vi "r3_stave HDI measure shih v1.vi"() -> ()   [LabVIEW 2016]
uses:
  <vilib>/Utility/file.llb/Read Delimited Spreadsheet (DBL).vi
  <vilib>/Utility/file.llb/Write Delimited Spreadsheet (DBL).vi
  Classes/Controllers/Motion/Copy of Motion Folder/Motion.lvclass
  Classes/Controllers/Camera/Copy of Controller Folder/Controller.lvclass
panel:
  in  "south - bottom right":bool
  in  "south - bottom left":bool
  in  "south - upper left":bool
  in  "north - bottom right":bool
  in  "north - bottom left":bool
  in  "north - upper left":bool
  out "txt check":dbl[][](array[numeric])
  in  "north first switch":bool
  out "position from OGP all":dbl[][][](array[numeric]) format="%#_8g"
  out "HDI-stave deviation all":dbl[][][](array[numeric]) format="%#_8g"
  out "HDI - stave deviation on time":dbl[][](array[numeric]) format="%#_8g"
  out "position from OGP on time":dbl[][](array[numeric]) format="%#_8g"
  in  "default south HDI upper left":dbl[](array[numeric])=[589.61399, 909.79853, 66.641535, 0.0001909297]
  in  "test":bool
  in  "how much HDI":i32=2
  out "bottom right":dbl[][](array[numeric]) format="%#_8g"
  out "bottom left":dbl[][](array[numeric]) format="%#_8g"
  out "top left":dbl[][](array[numeric]) format="%#_8g"
  out "HDI center position":dbl[][](array[numeric]) format="%#_8g"
  in  "default north HDI upper left":dbl[](array[numeric])=[589.67627, 676.52803, 66.636955, 0.0001904]
  in  "Default HDI size":dbl[](array[numeric])=[24.2437, 231.446, -0.099339, 0.000191129]
  out "measure times":dbl
  in  "Parking position":dbl[](array[numeric])=[625.0, 625.0, 0.0, 0.01]
  in  "measure HDI position":bool
  in  "calculate":bool
  in  "go to park":bool
  in  "stop":bool
  # "Please click the \"make north first\" before calculate\nIf there is new txt from \"Bless from OGP\", please click \"make north first\", then click the \"calculate\""
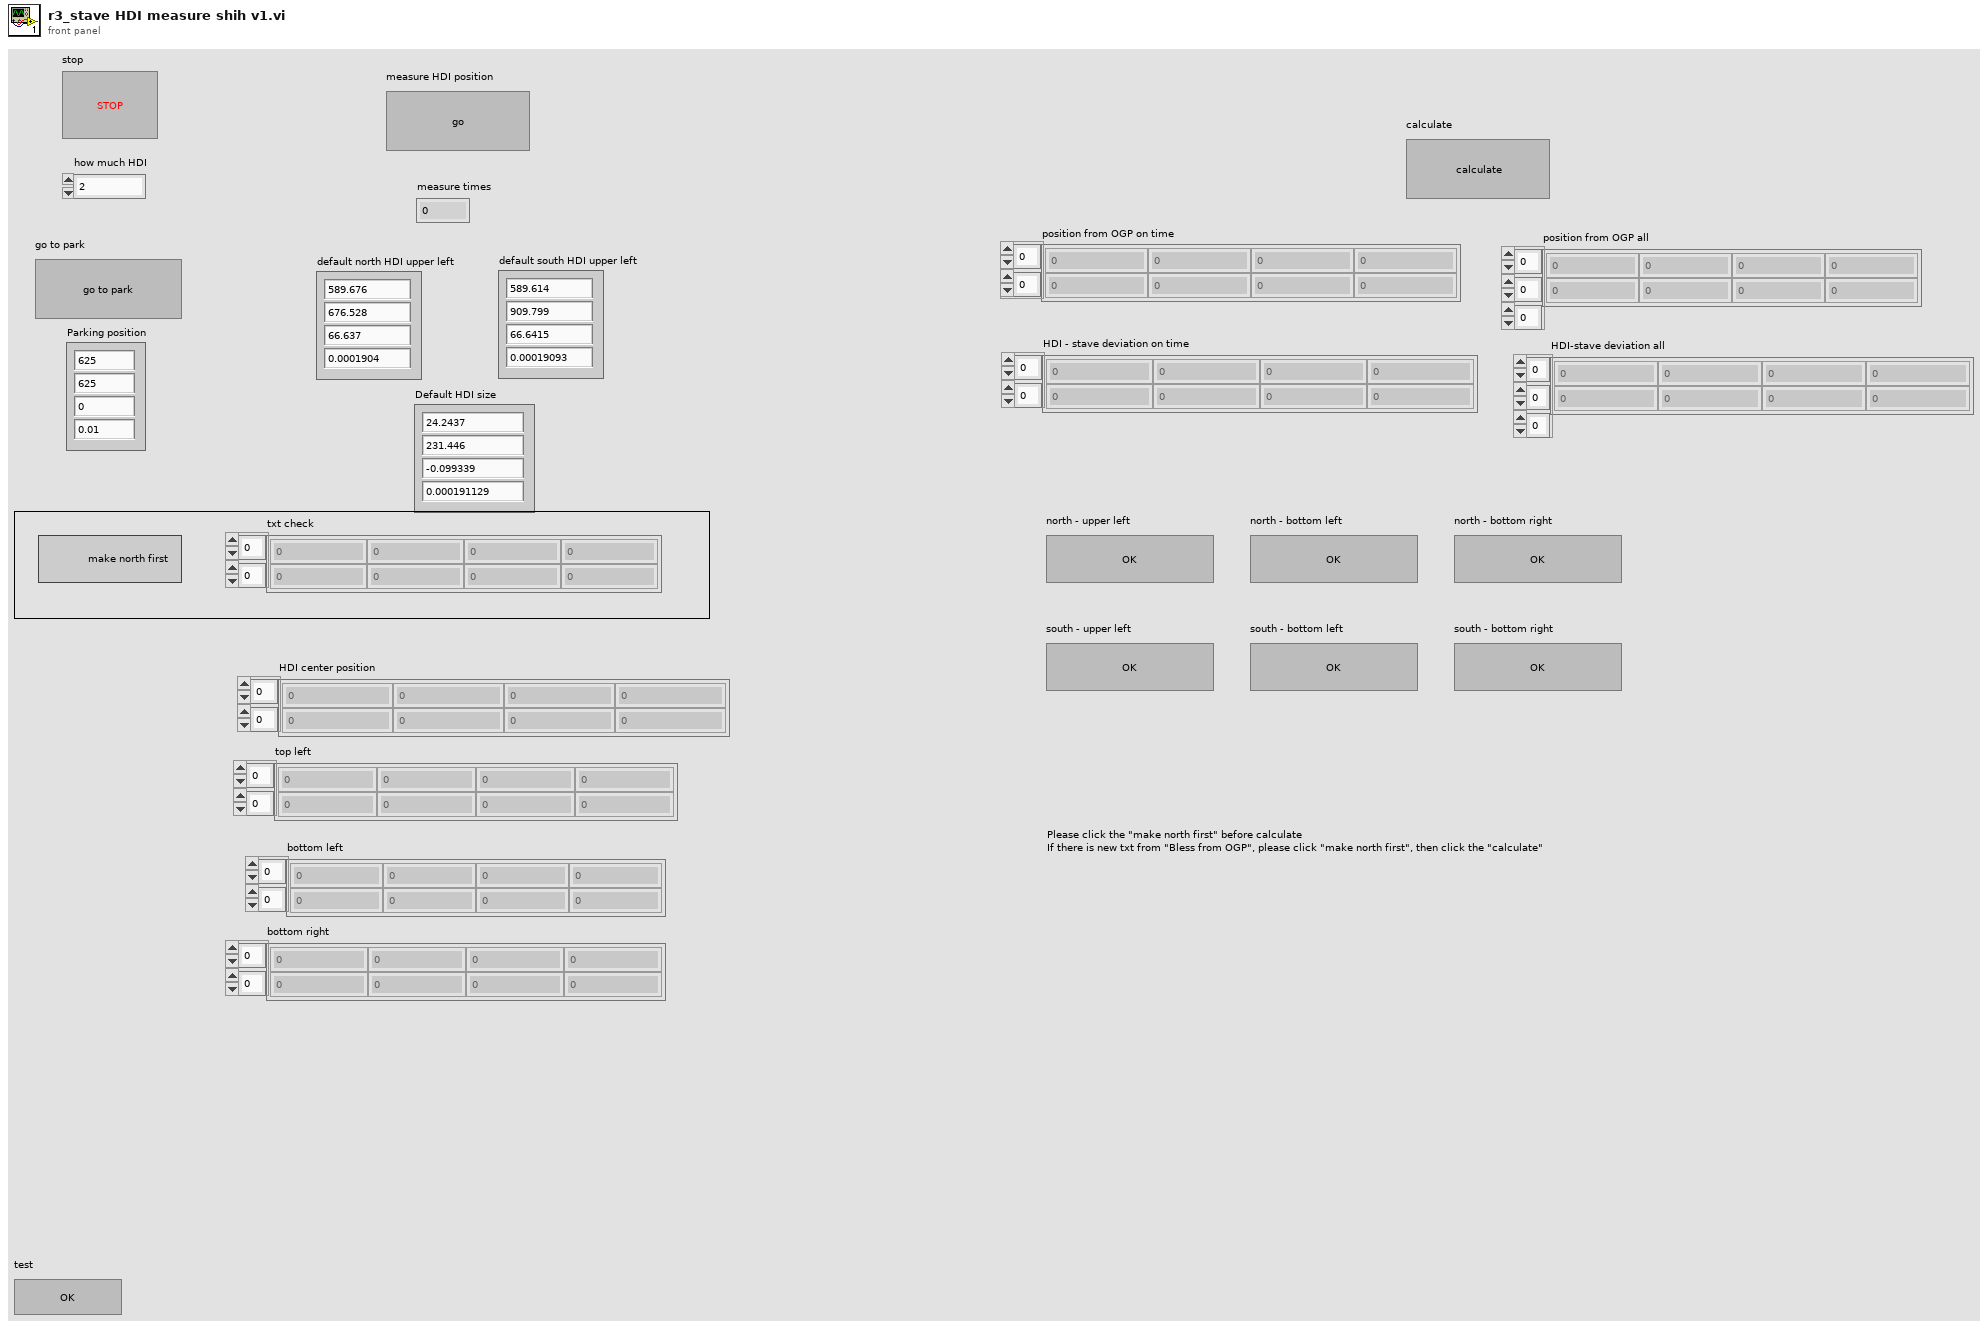
[diagram p1: front panel]
types:
  T1 = typedef "Controller.lvclass/Controllers.ctl" = cluster{"Copy of Motion.lvclass":refnum<class "Motion.lvclass">, "Copy of I-O.lvclass":refnum<class "I-O.lvclass">, "Copy of Dispenser.lvclass":refnum<class "Dispenser.lvclass">}
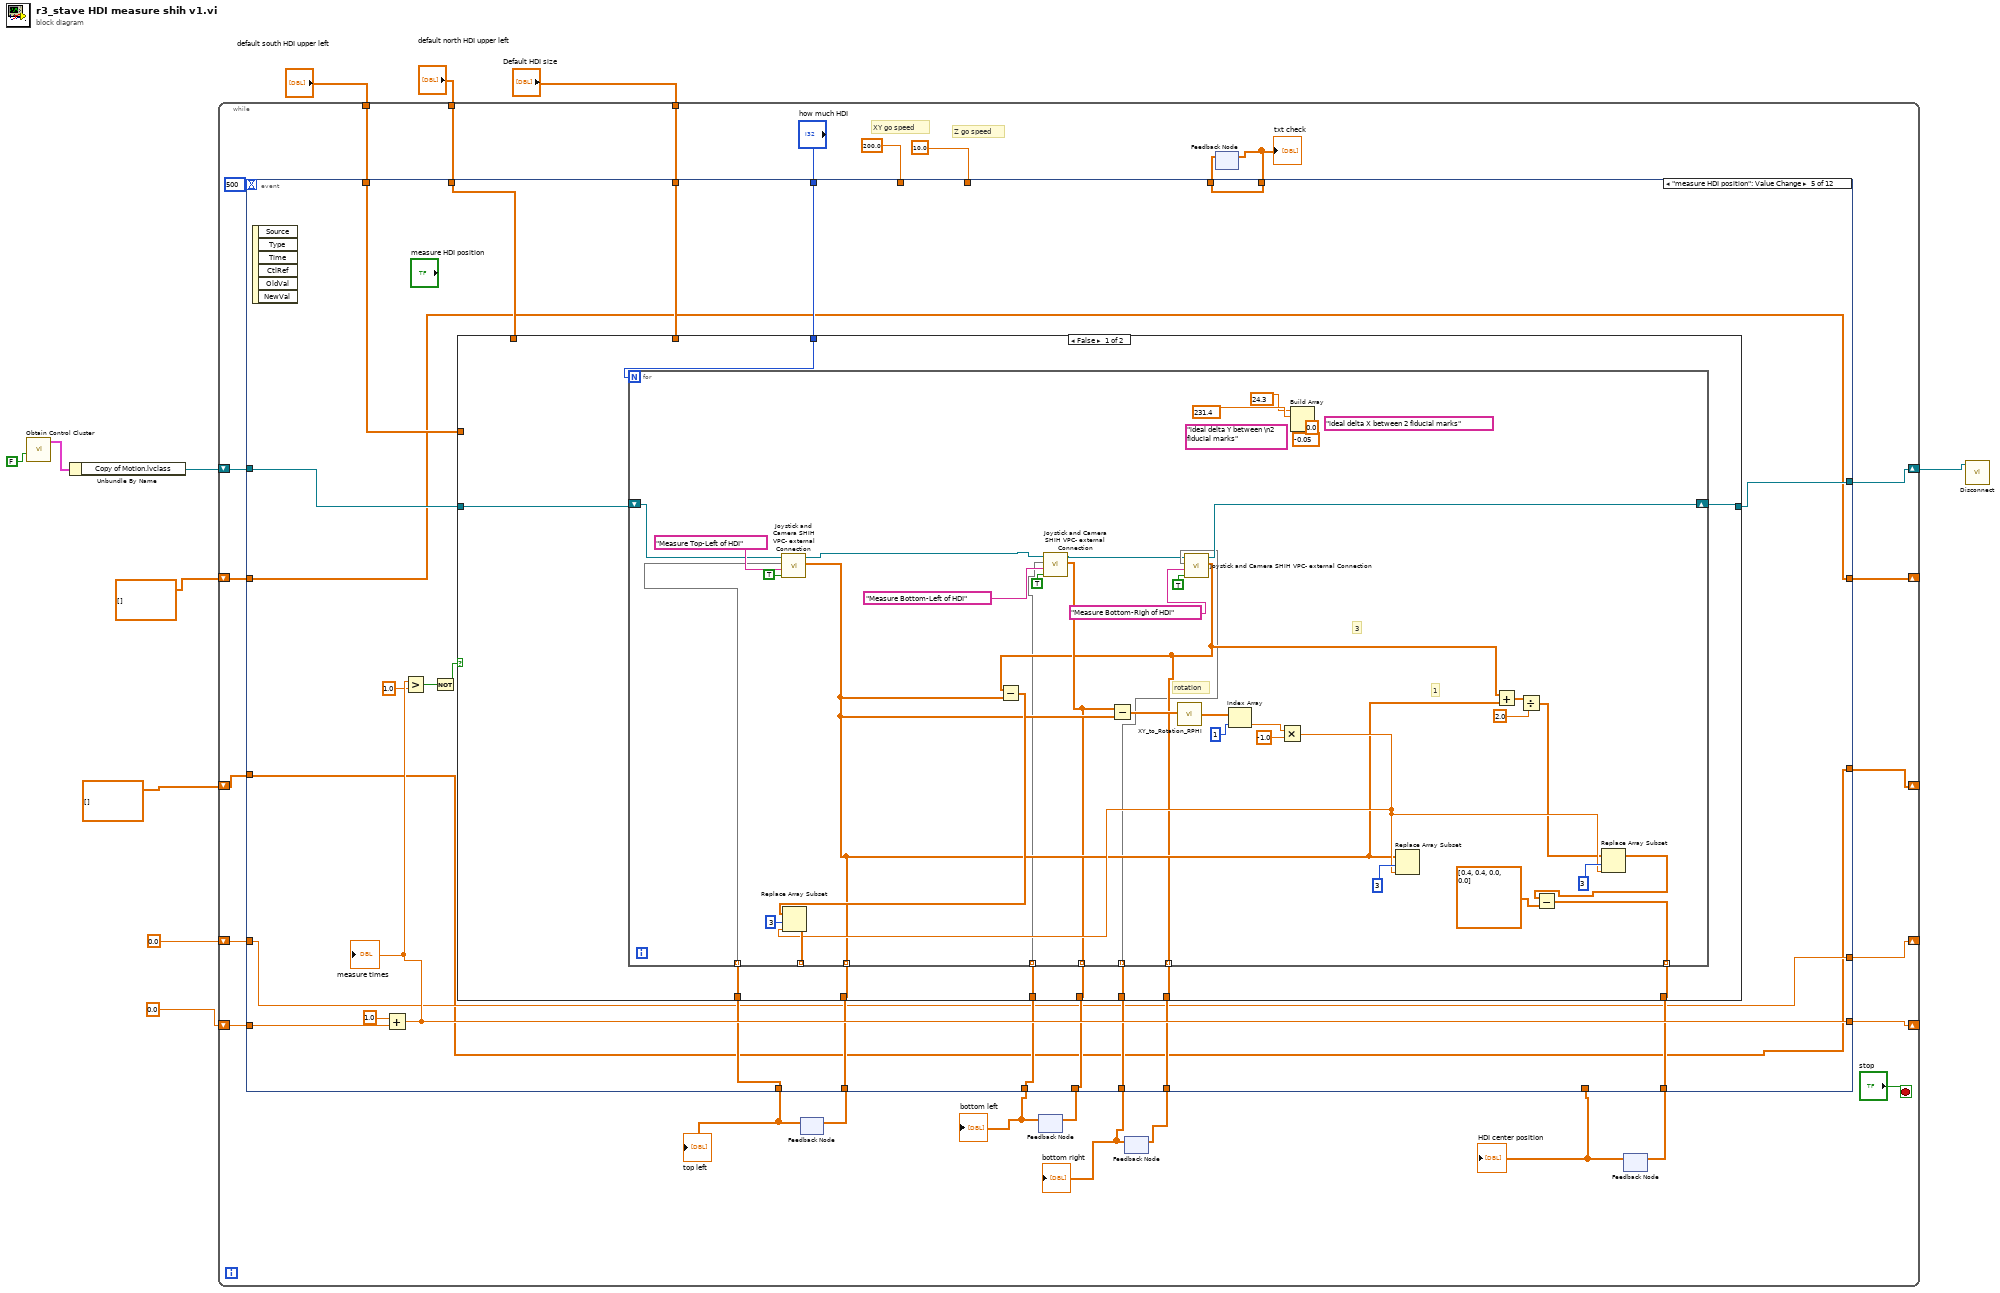
[diagram p0: block diagram]
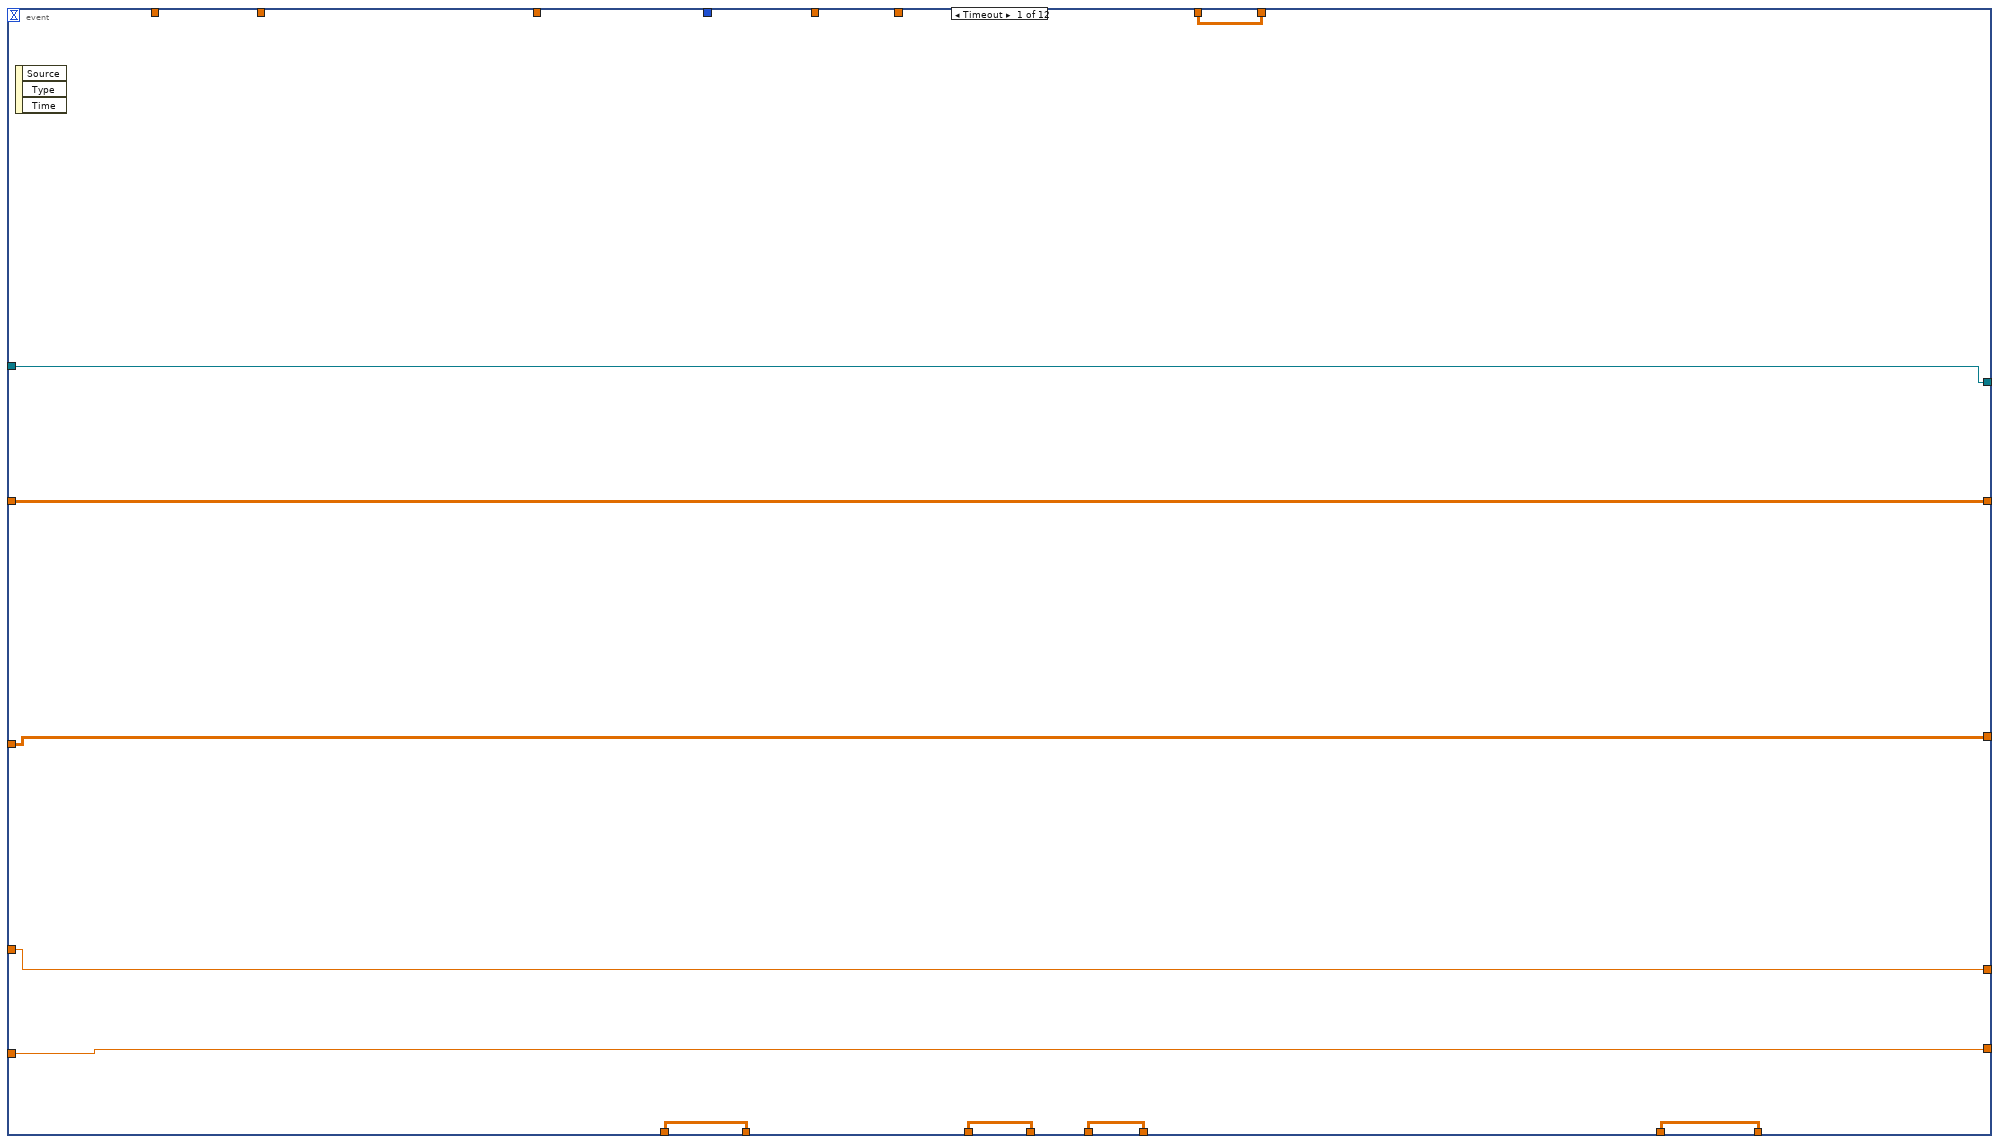
[diagram p2: hidden frame]
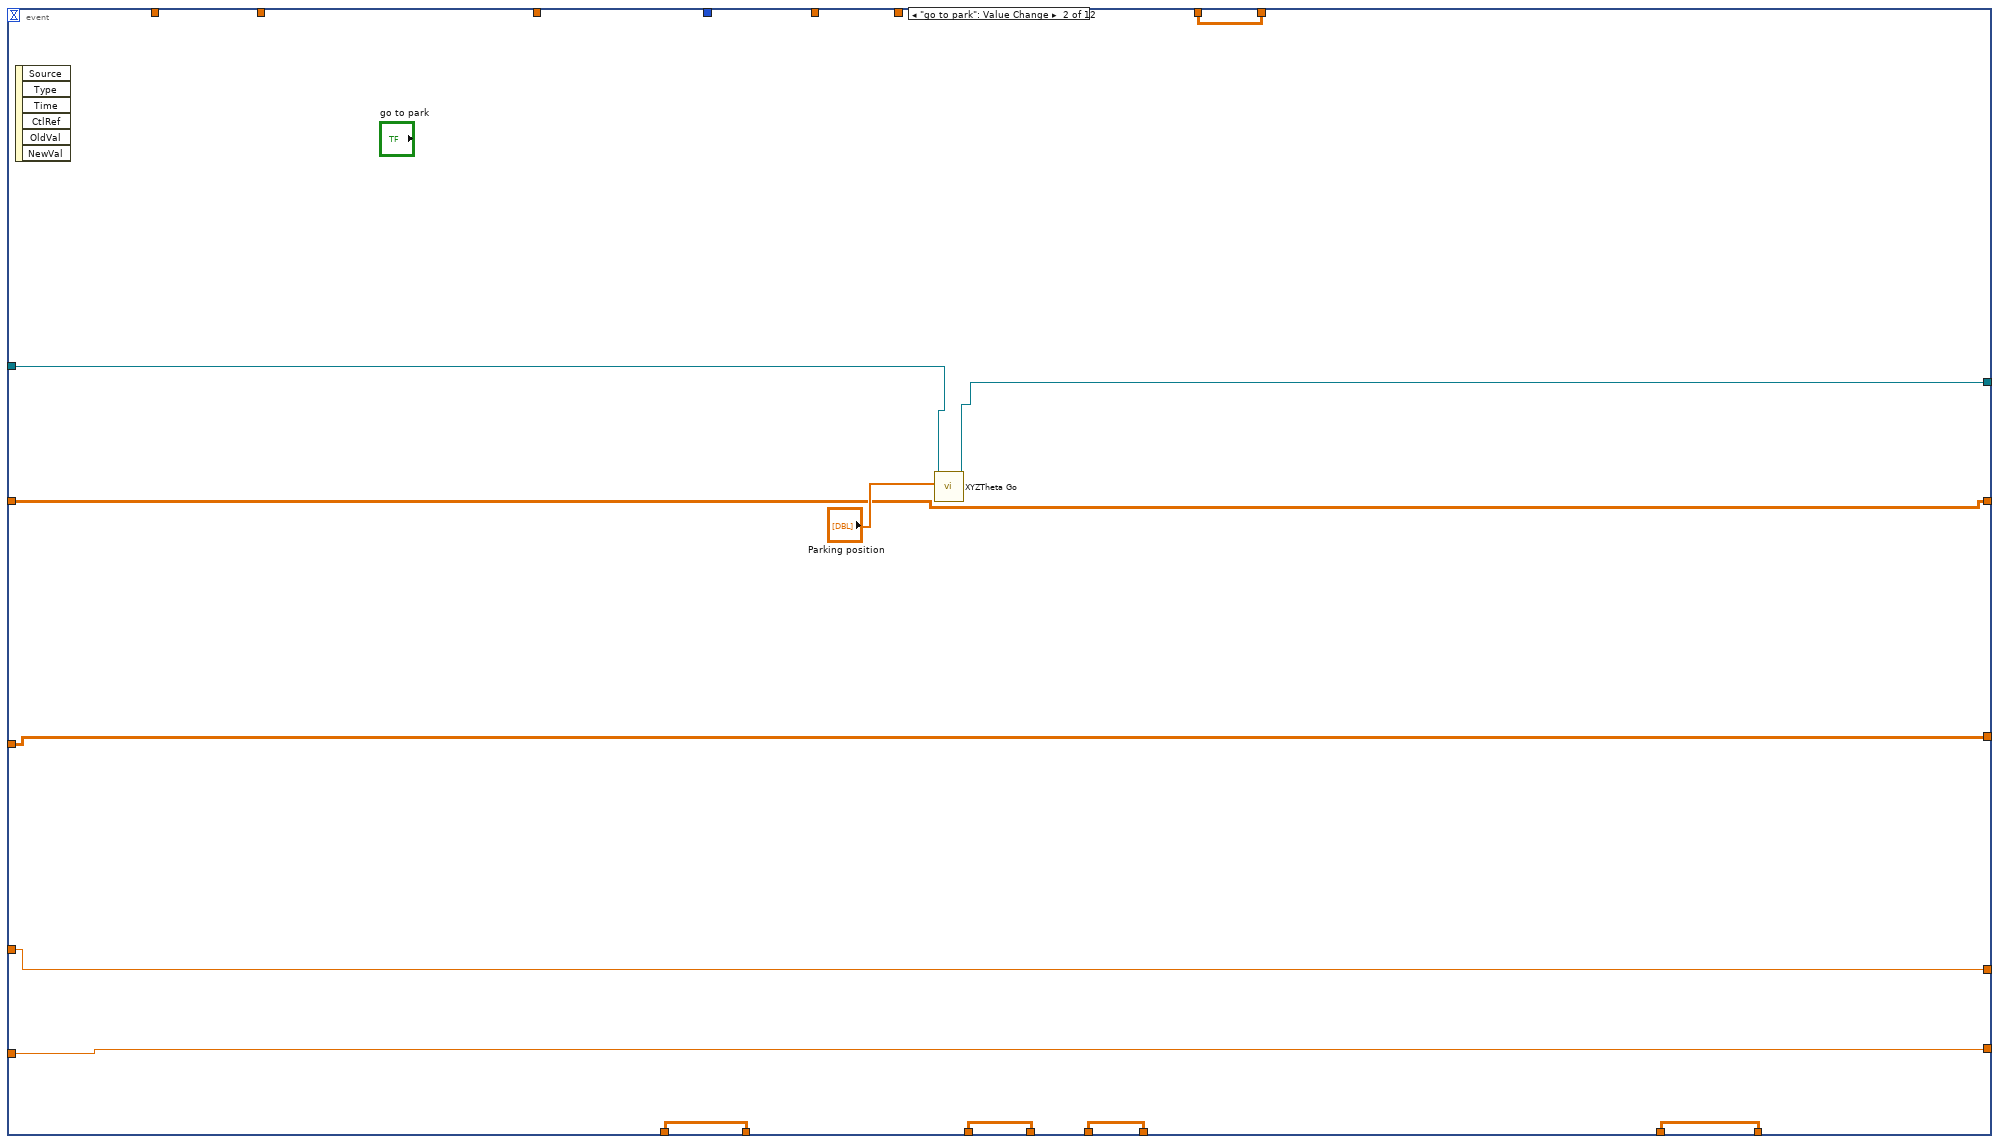
[diagram p3: hidden frame]
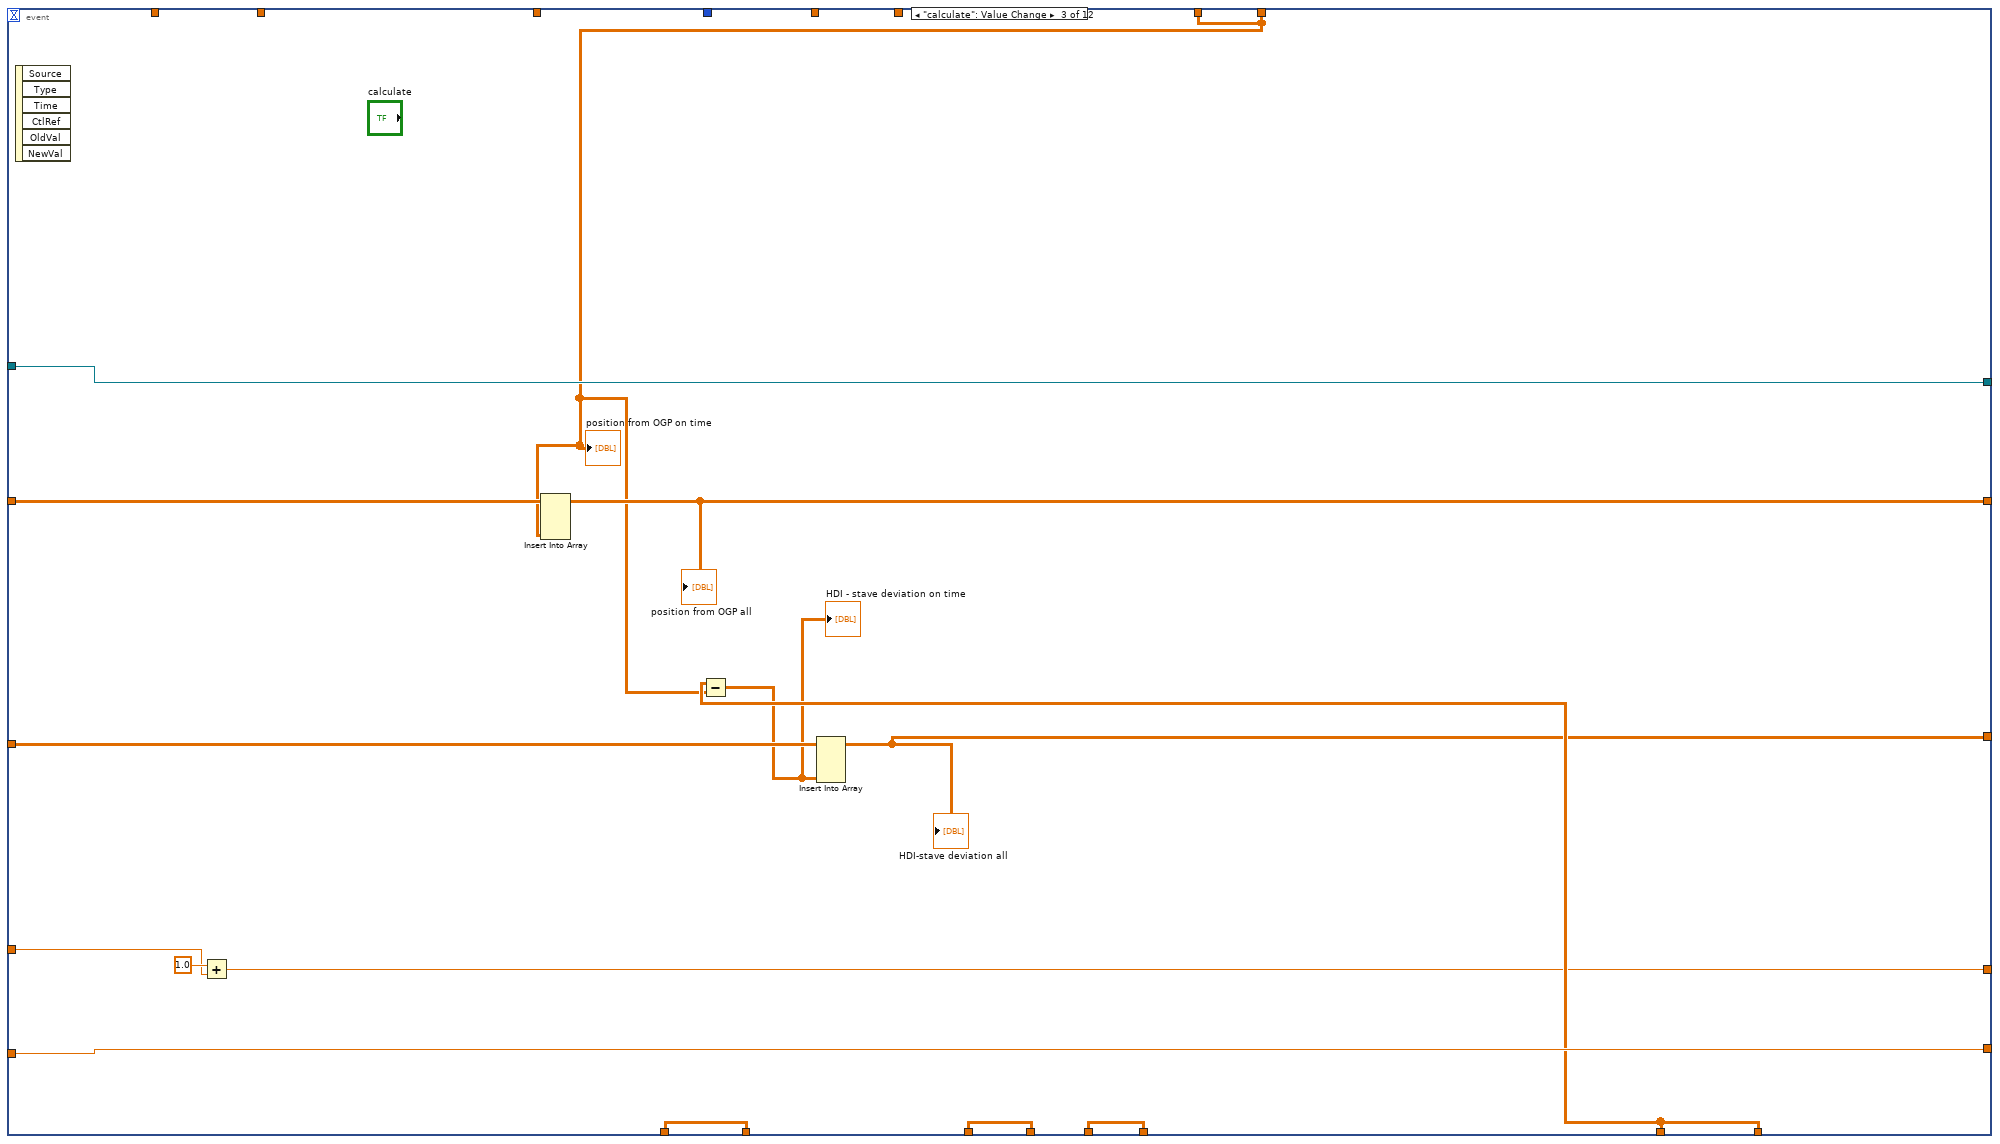
[diagram p4: hidden frame]
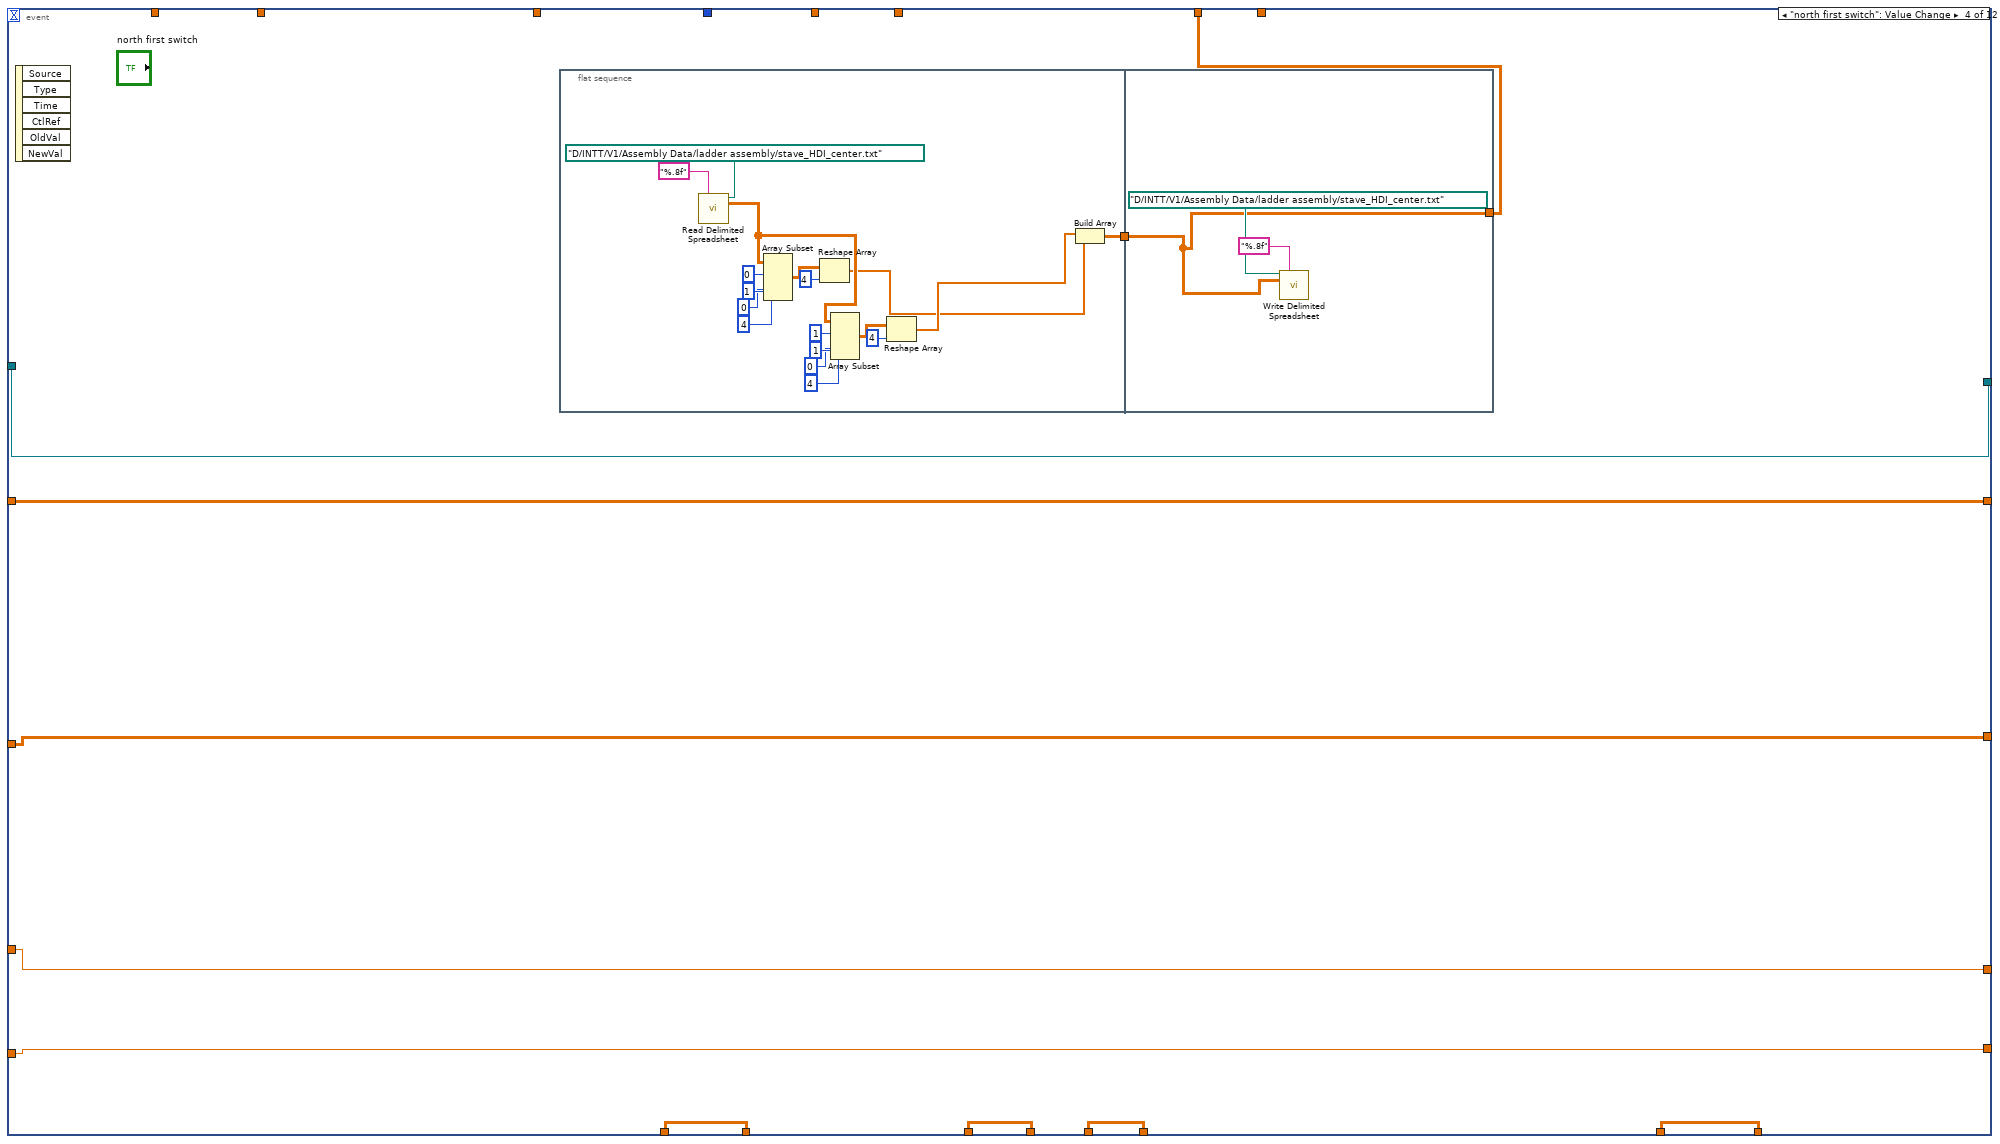
[diagram p5: hidden frame]
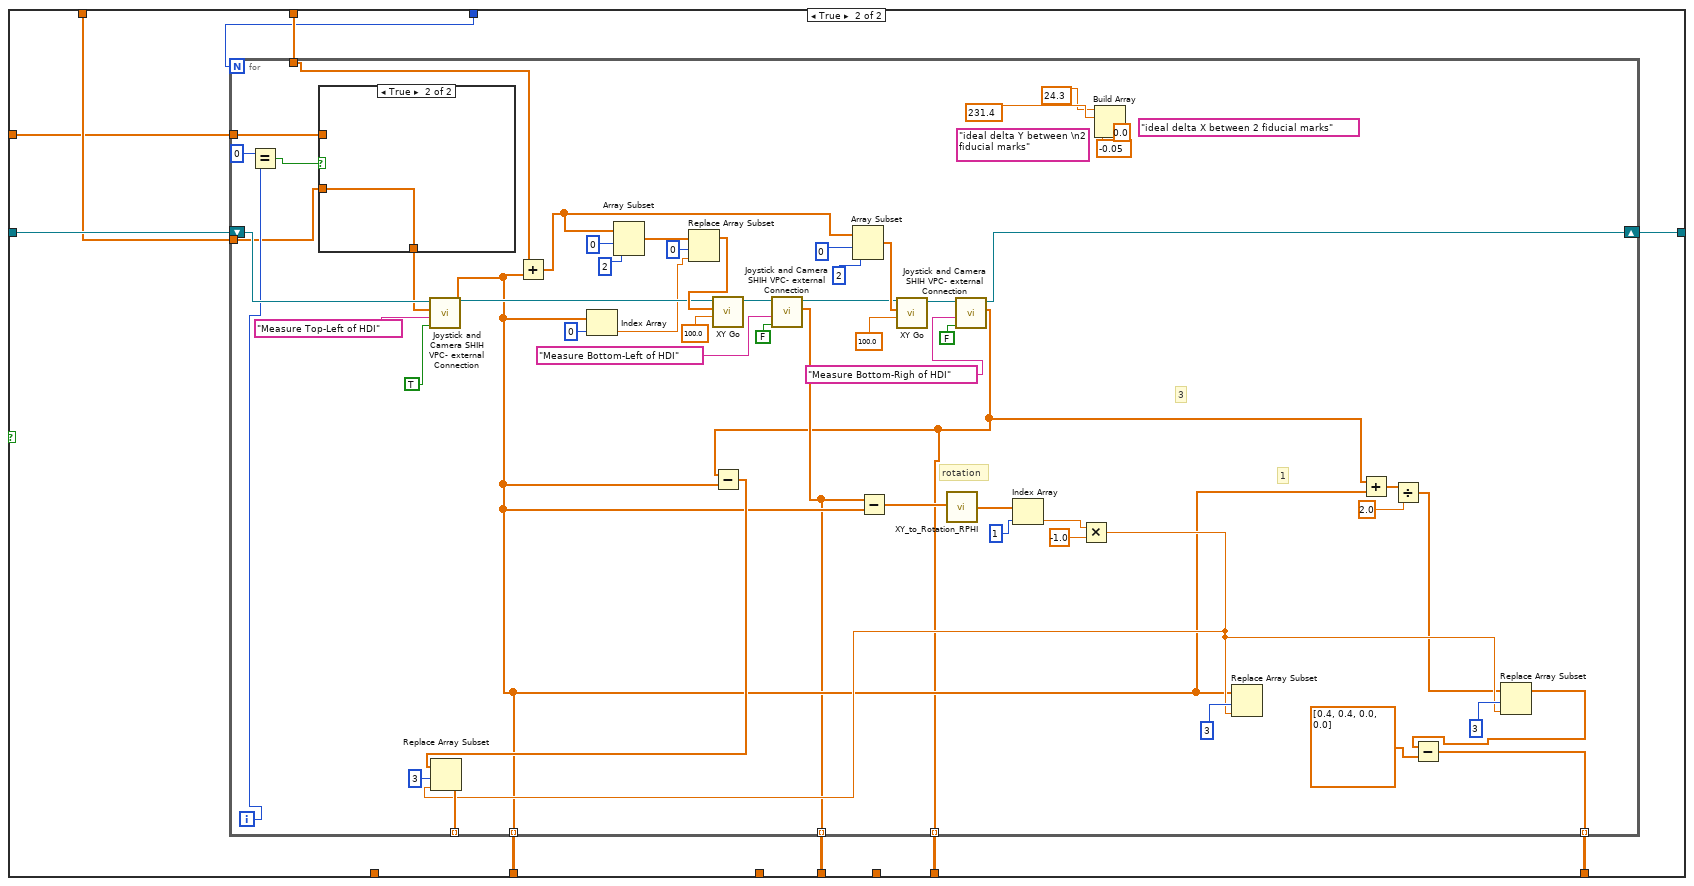
[diagram p6: hidden frame]
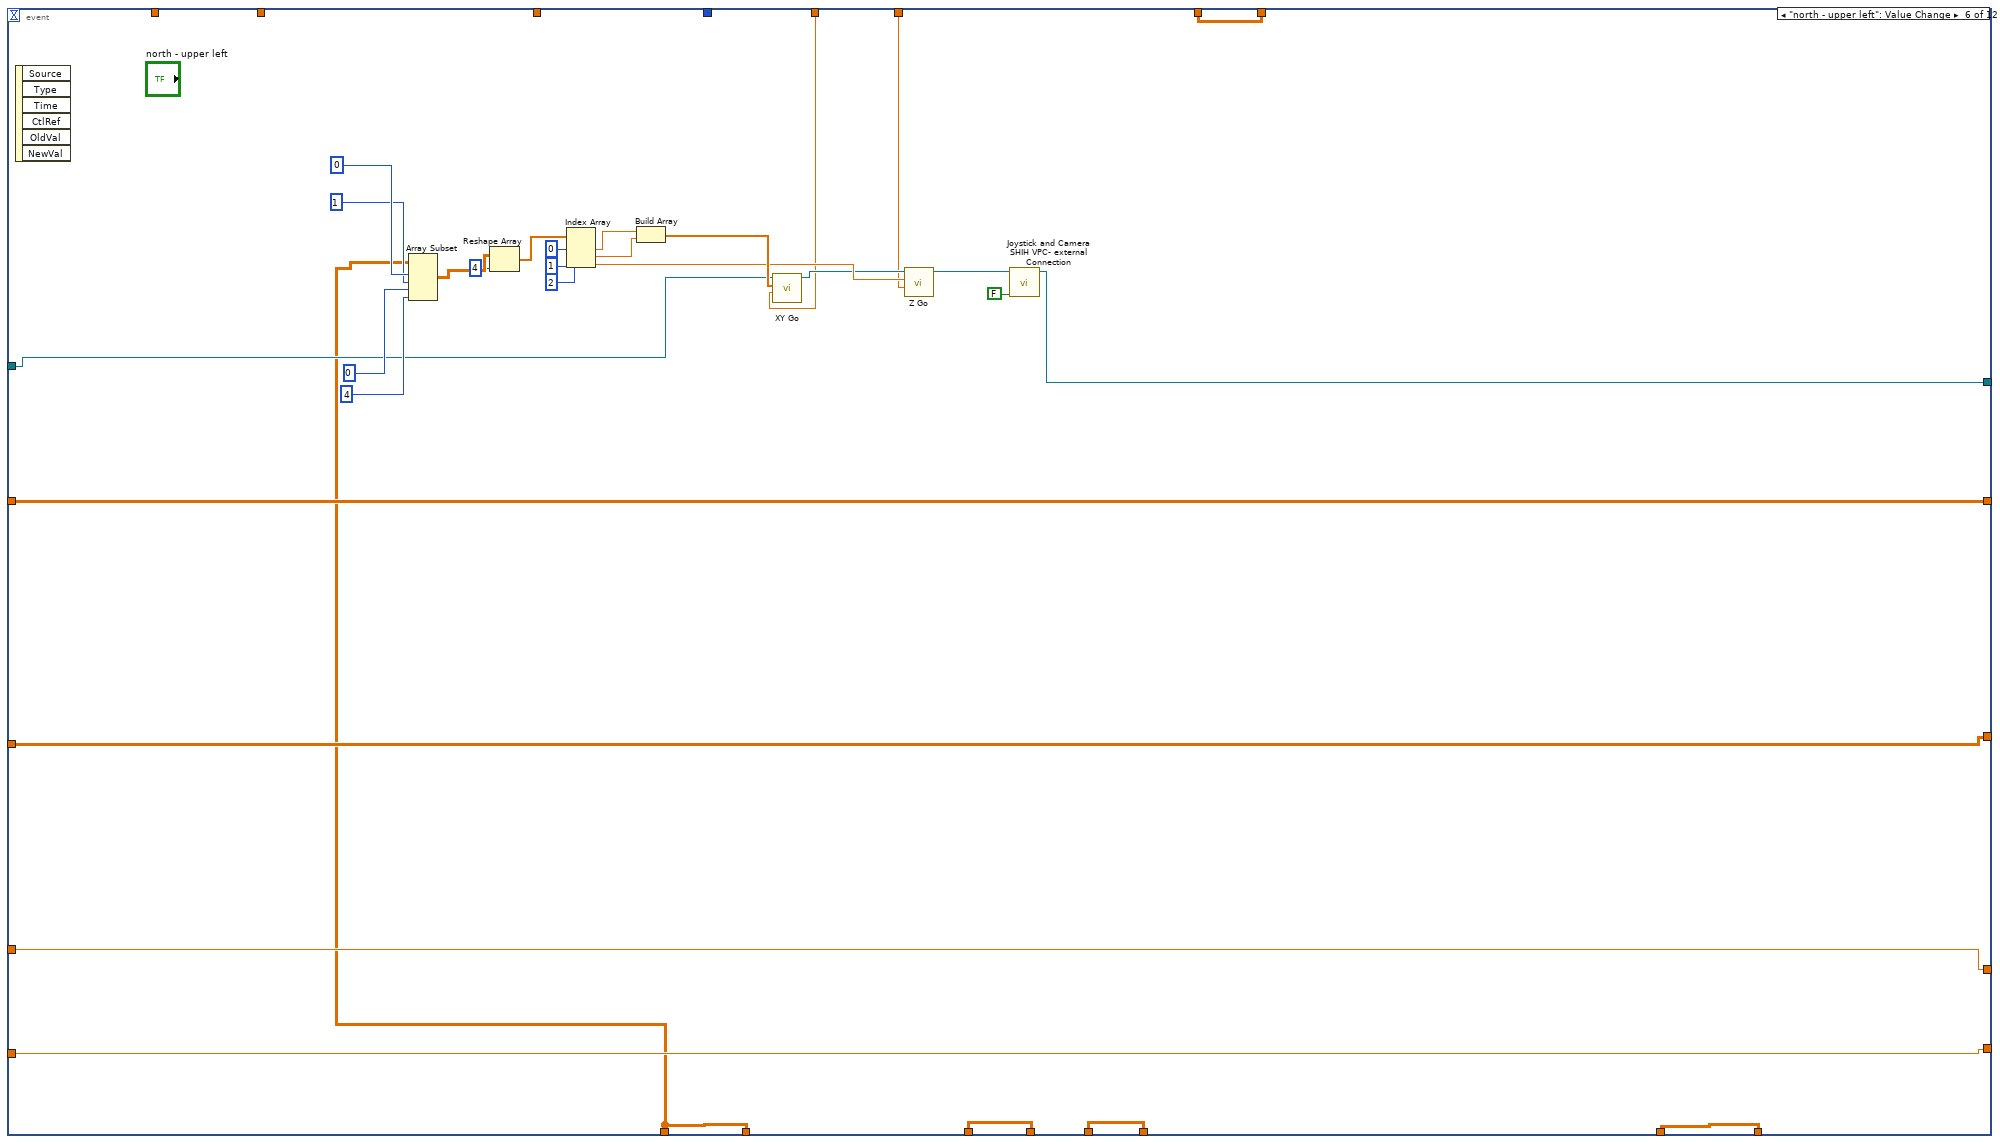
[diagram p8: hidden frame]
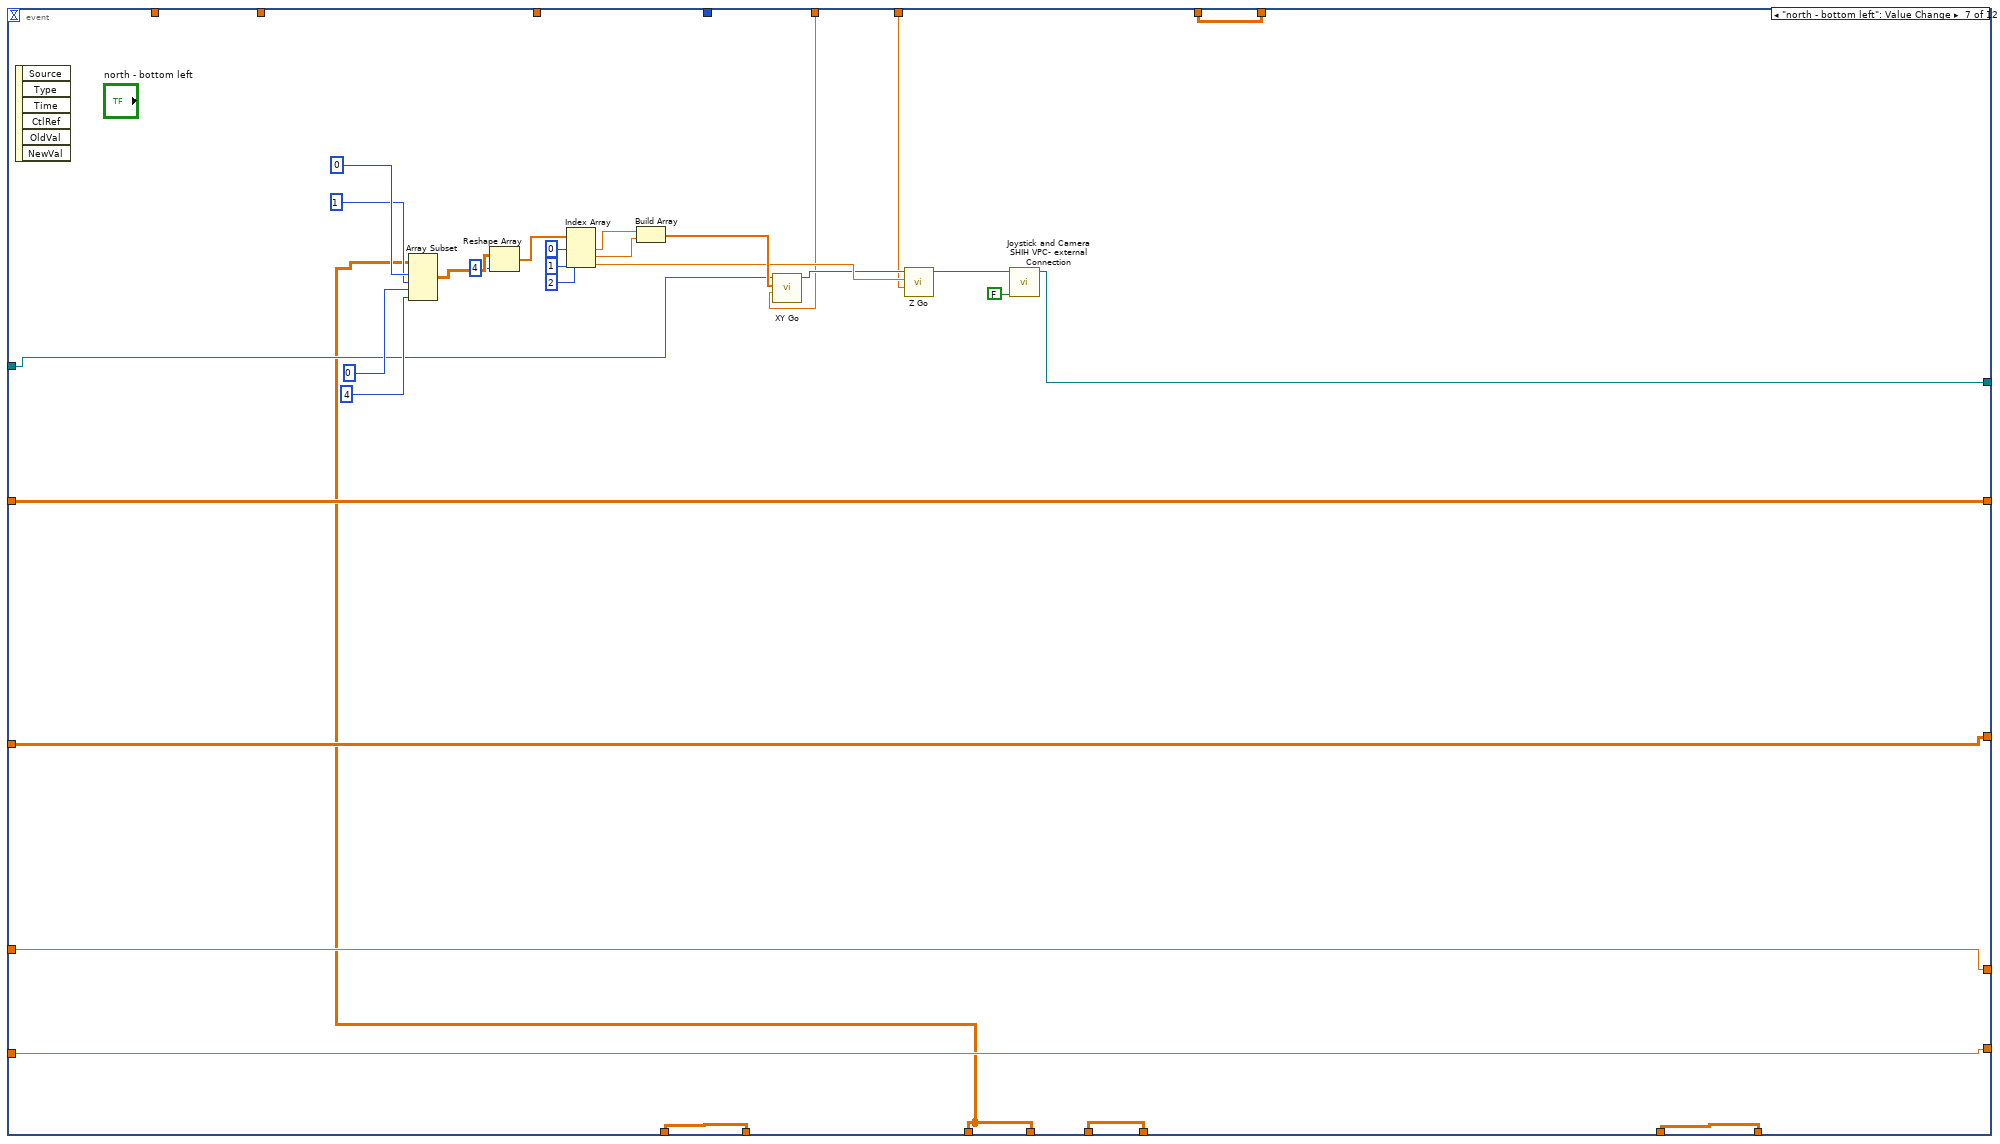
[diagram p9: hidden frame]
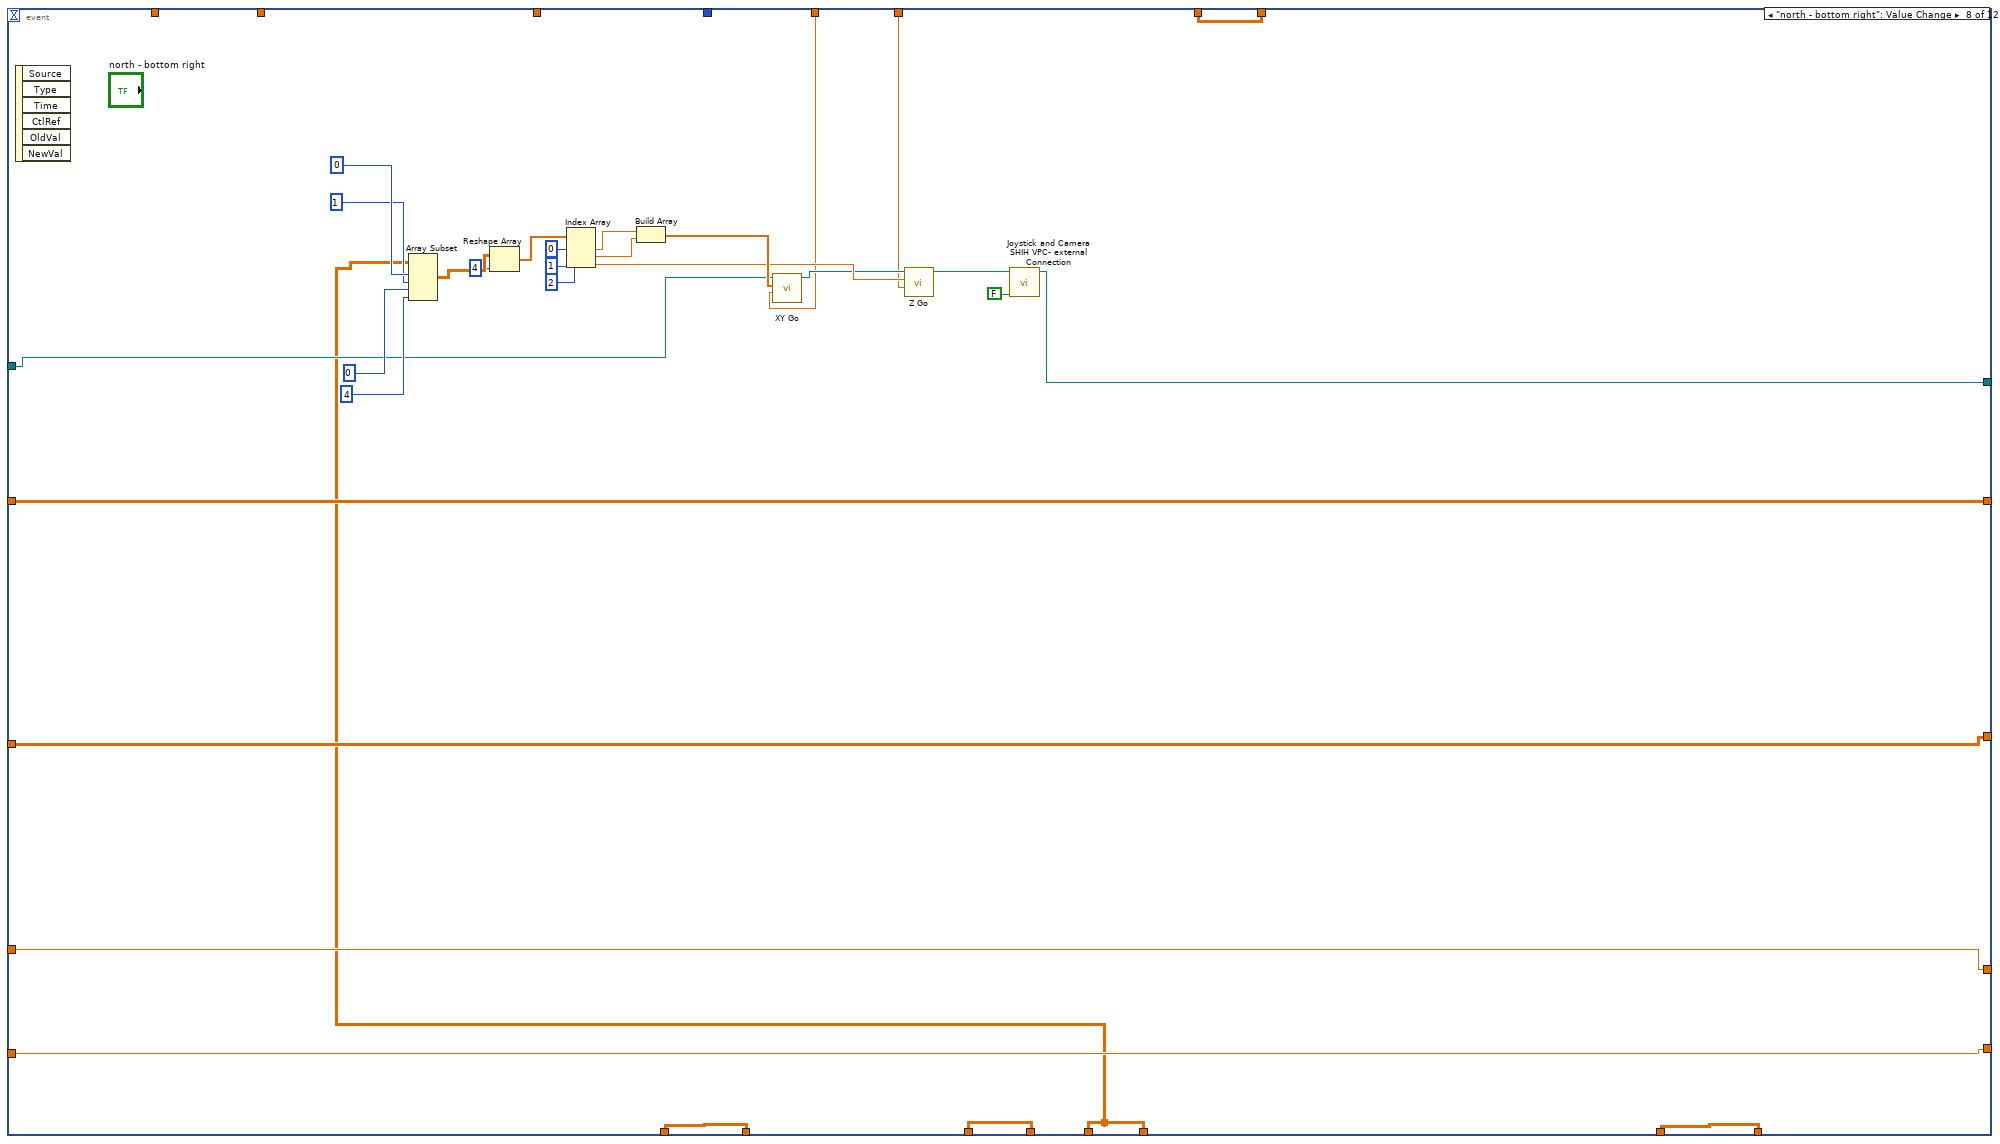
[diagram p10: hidden frame]
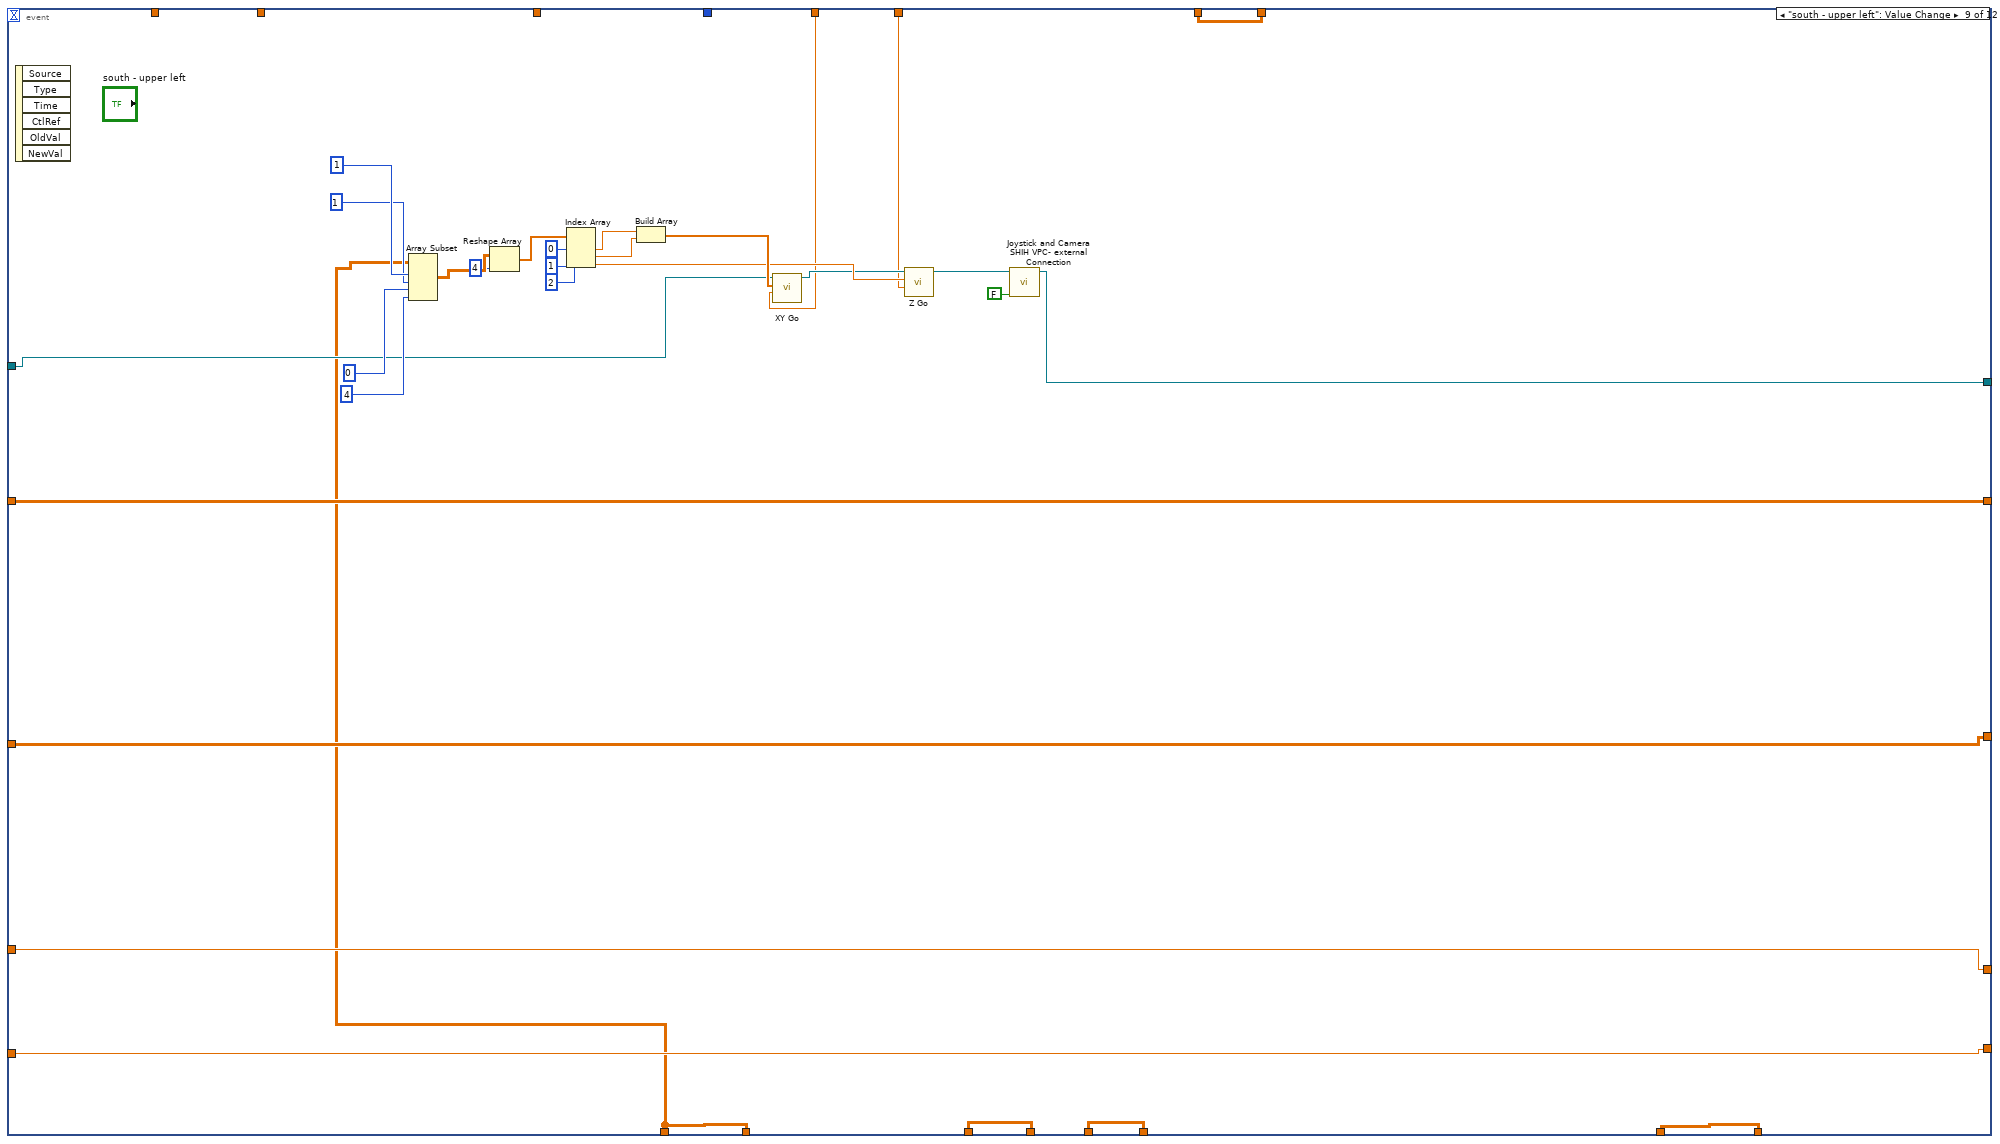
[diagram p11: hidden frame]
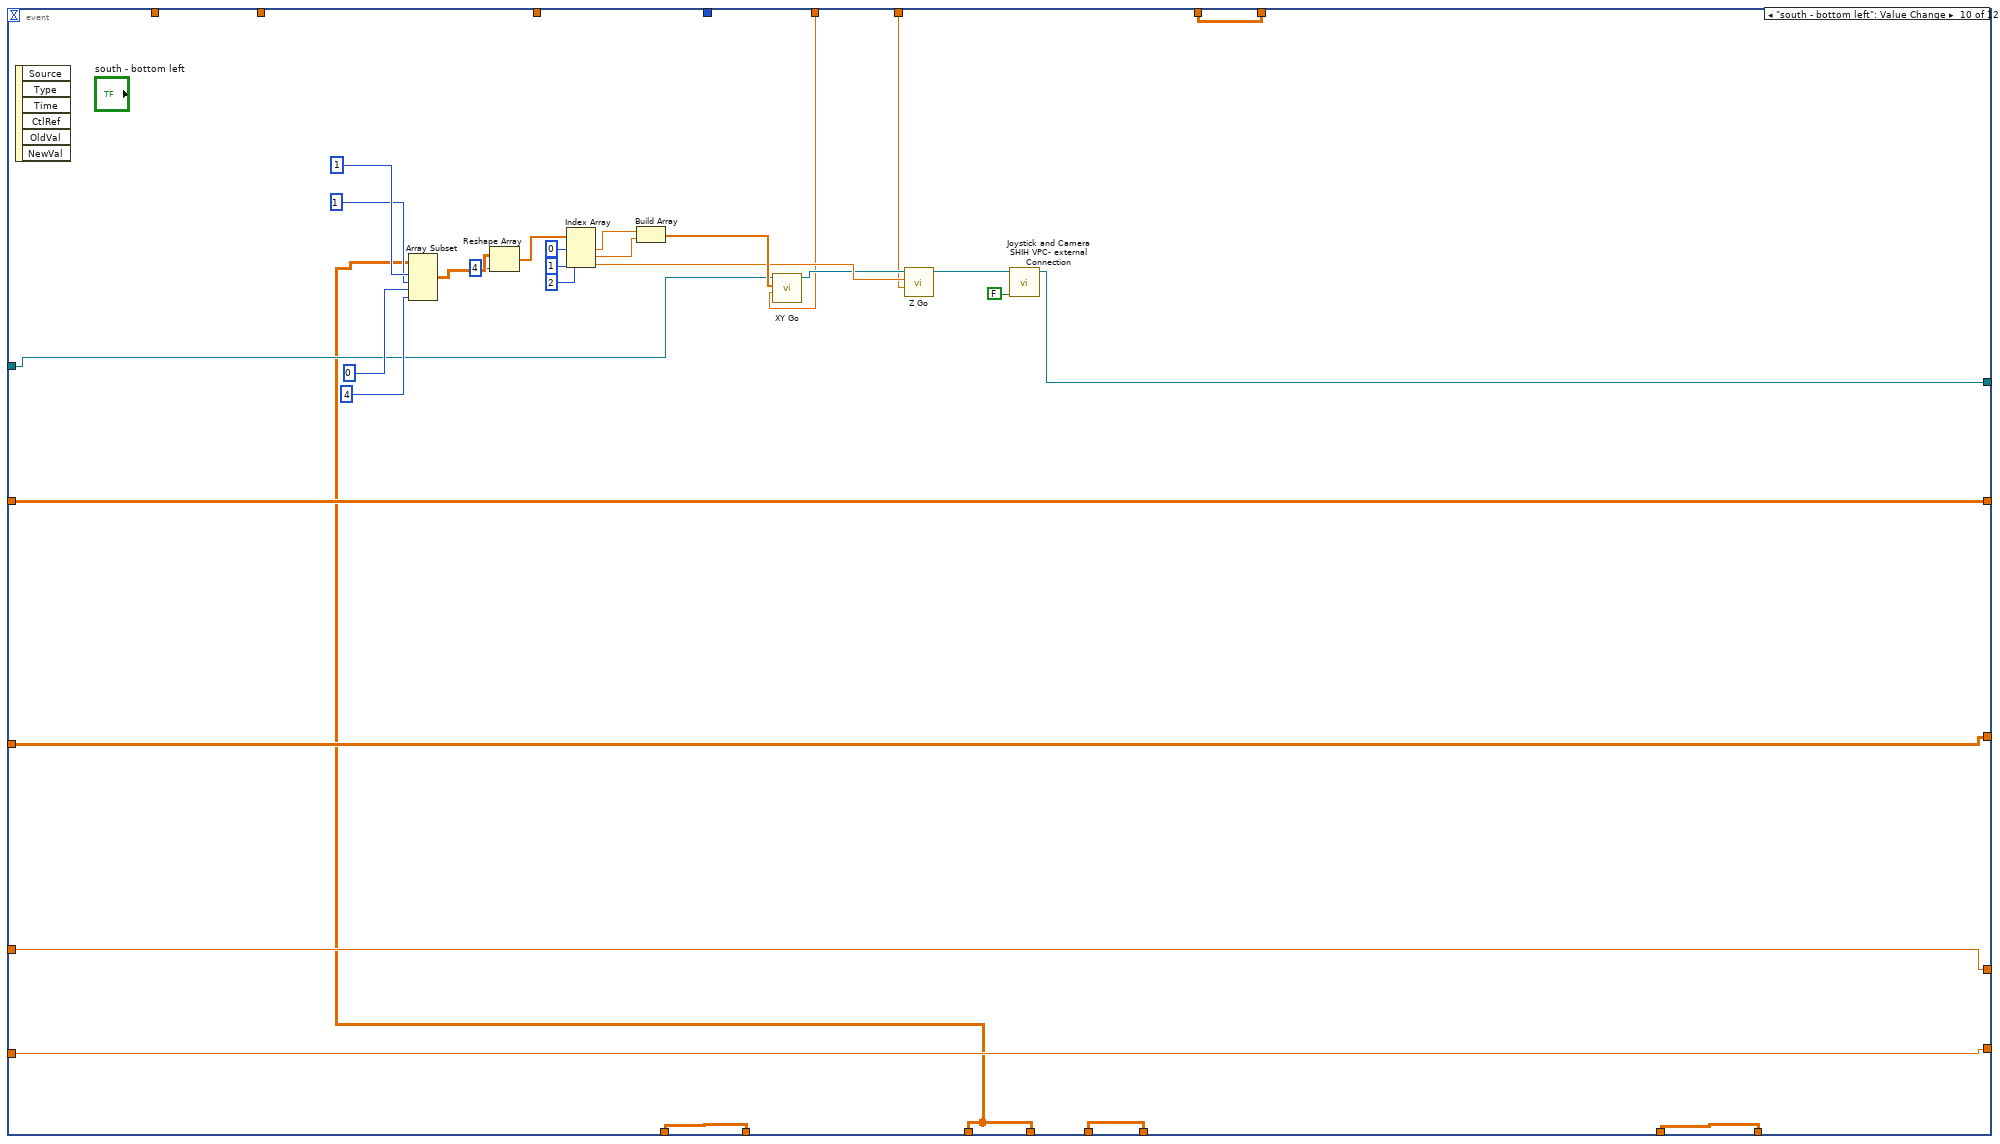
[diagram p12: hidden frame]
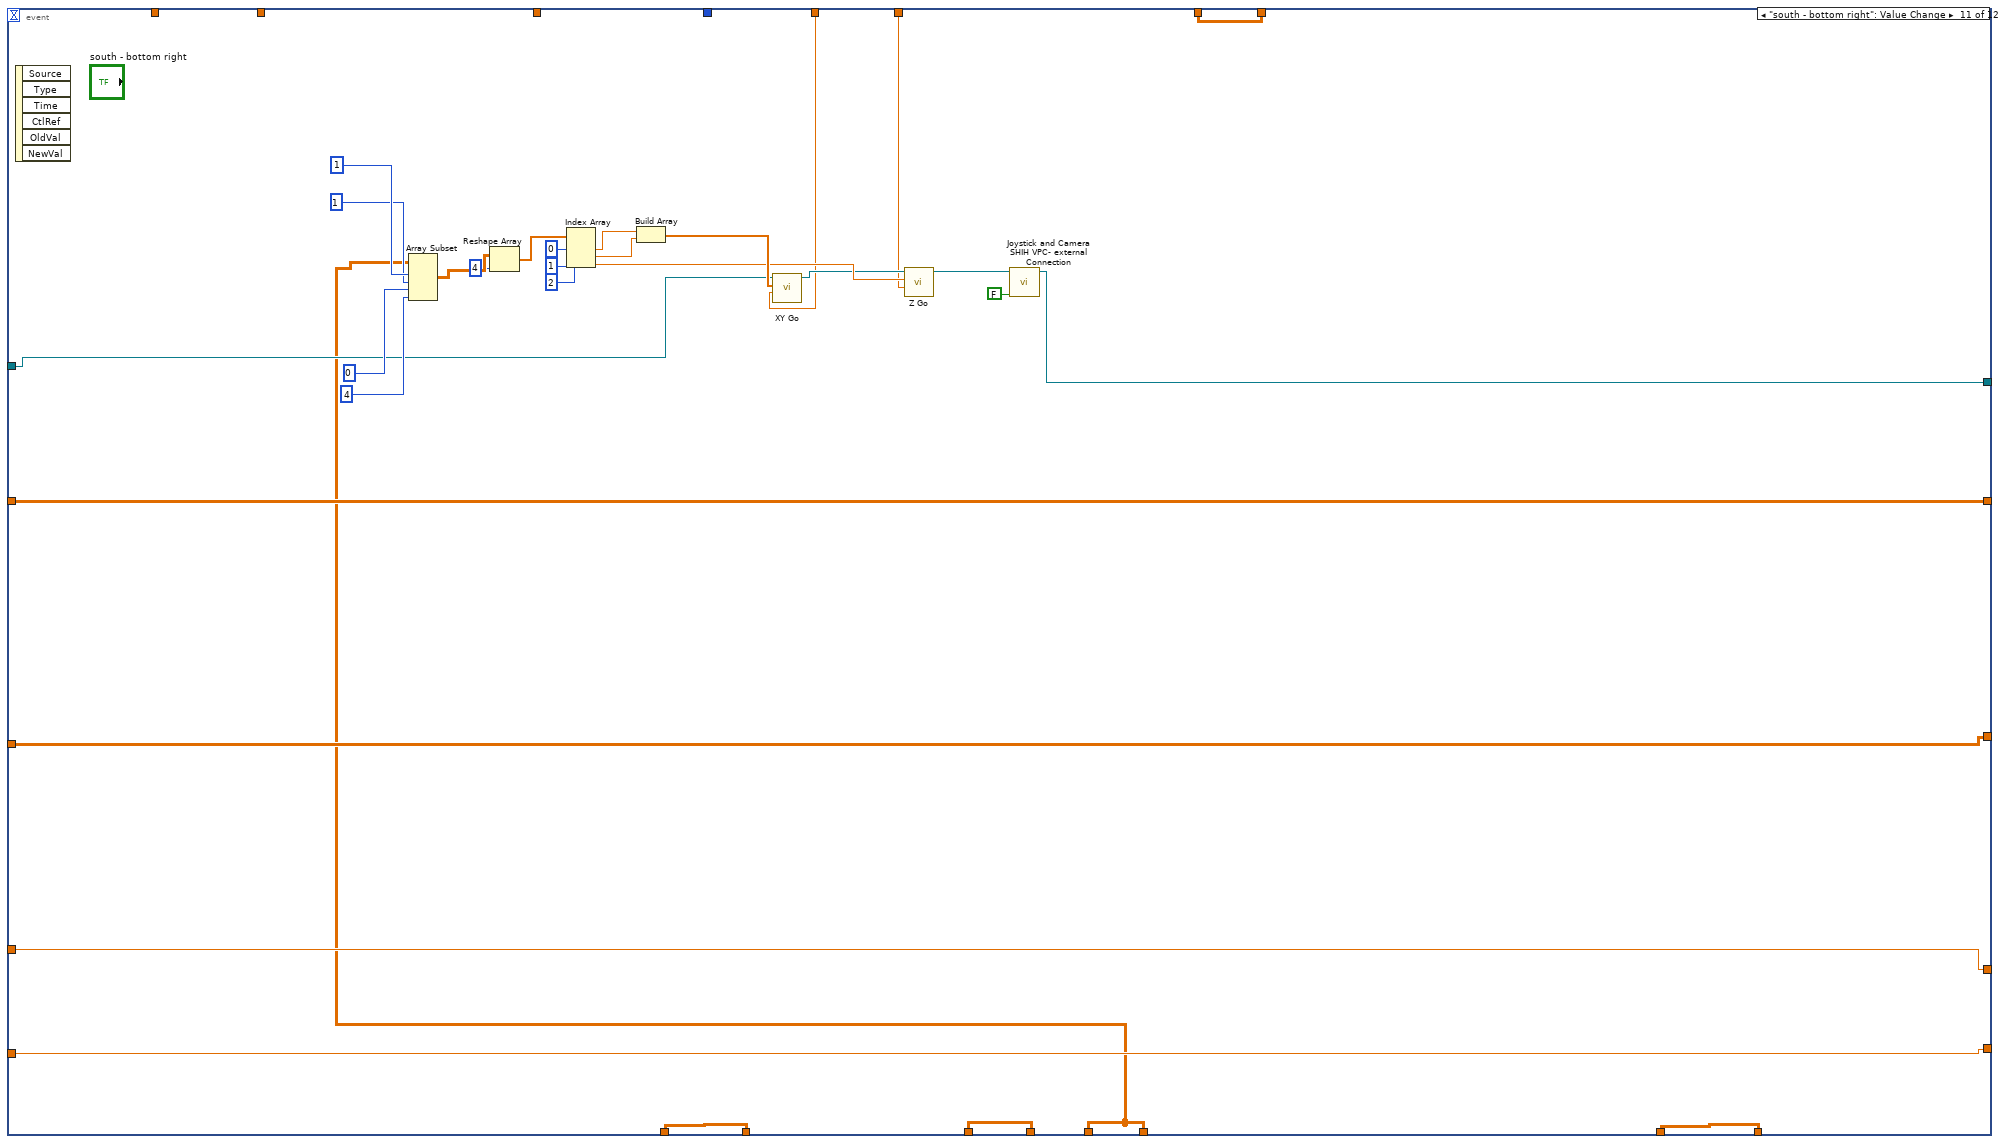
[diagram p13: hidden frame]
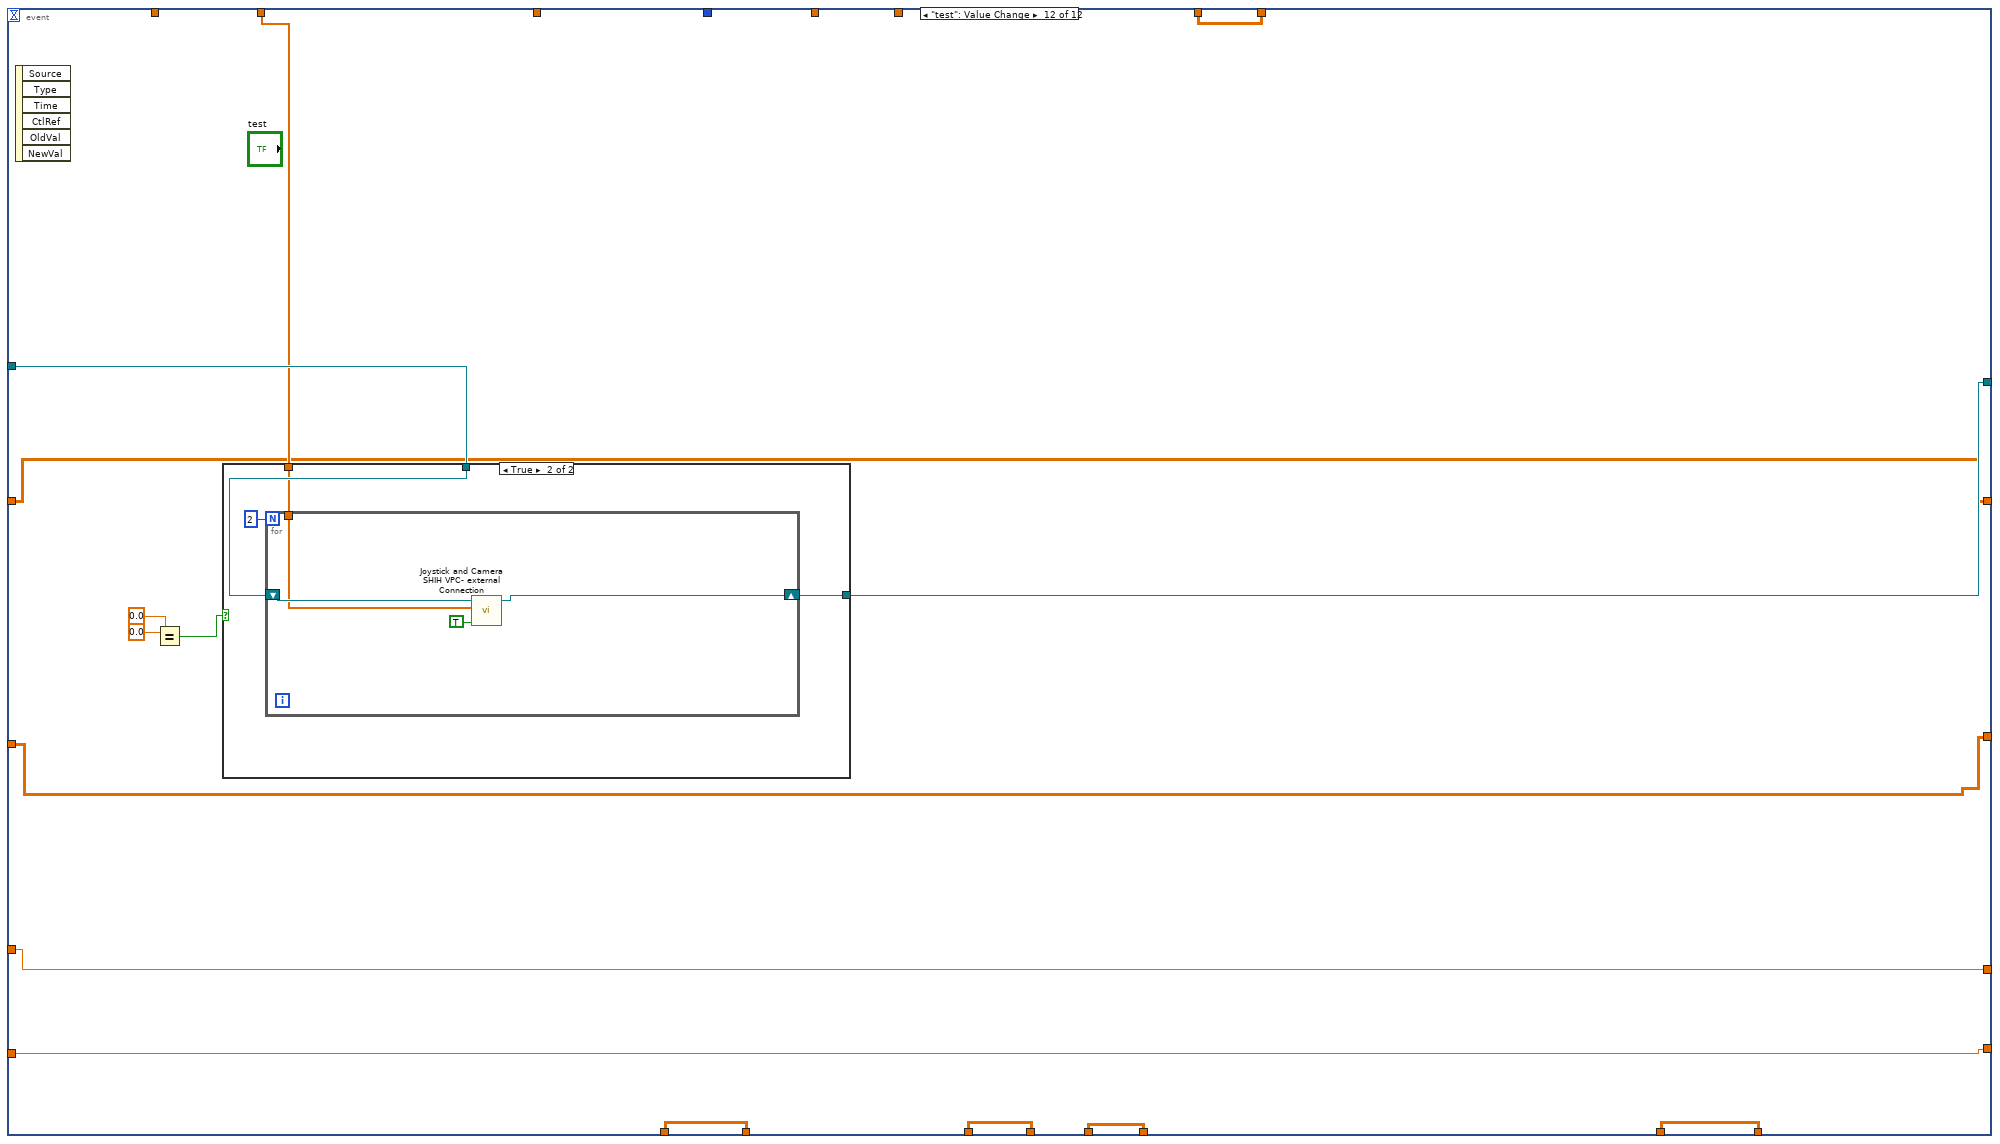
[diagram p14: hidden frame]
diagram:
  n1 = call "Obtain Control Cluster.vi"("I/O"=FALSE) -> ("Control Out"=w11:T1)  [unwired: 10 in]
  n2 = Unbundle By Name(w11) -> ("Copy of Motion.lvclass"=w9:refnum<class "Motion.lvclass">)
  n3 = while {
    shift-right: [w36] -> w8
    shift-left: w9 -> [w37]
    shift-right: [w34] -> _
    shift-left: 0.0 -> [w35]
    tunnel: "Default HDI size" -> [w33]
    tunnel: "default north HDI upper left" -> [w32]
    tunnel: "default south HDI upper left" -> [w23]
    shift-right: [w20] -> _
    shift-left: 0.0 -> [w21]
    shift-right: [w18] -> _
    shift-left: dbl[][][] [] -> [w19]
    shift-right: [w16] -> _
    shift-left: dbl[][][] [] -> [w17]
    stop <- "stop" stop-if-true
    # "Z go speed"
    # "XY go speed"
    n4 = feedback #1() -> (w29:dbl[][])  [unwired: 1 in]
    "top left" <- w29
    n5 = feedback #2() -> (w26:dbl[][])  [unwired: 1 in]
    "bottom left" <- w26
    n6 = feedback #3() -> (w25:dbl[][])  [unwired: 1 in]
    "bottom right" <- w25
    n7 = feedback #4() -> (w14:dbl[][])  [unwired: 1 in]
    "txt check" <- w14
    n8 = feedback #5() -> (w22:dbl[][])  [unwired: 1 in]
    "HDI center position" <- w22
    n9 = event shown="[4] \"measure HDI position\": Value Change" {
      selector: _ -> [_ _ _ _ _ _ _ _ _ _ _ _]
      dyn-events: _ -> [_ _ _ _ _ _ _ _ _ _ _ _]
      timeout: 500 -> [_ _ _ _ _ _ _ _ _ _ _ _]
      tunnel: w37 -> [w49 w60 w76 w87 w131 w257 w287 w317 w347 w377 w407 w441]
      tunnel: [w49 w59 w76 w87 w115 w252 w282 w312 w342 w372 w402 w440] -> w36
      tunnel: w35 -> [w44 w54 w72 w83 w130 w275 w305 w335 w365 w395 w425 w439]
      tunnel: [w44 w54 w72 w83 w128 w275 w305 w335 w365 w395 w425 w439] -> w34
      tunnel: w33 -> [_ _ _ _ w124 _ _ _ _ _ _ _]
      tunnel: w32 -> [_ _ _ _ w123 _ _ _ _ _ _ w438]
      tunnel: [w48 w58 w71 w79 w122 w249 w280 w310 w339 w370 w400 w431] -> w31
      tunnel: w22 -> [w48 w58 w71 w79 _ w249 w280 w310 w339 w370 w400 w431]
      tunnel: [w47 w57 w75 w82 w121 w248 w279 w309 w338 w369 w399 w434] -> w30
      tunnel: w29 -> [w47 w57 w75 w82 w118 w248 w279 w309 w338 w369 w399 w434]
      tunnel: [w46 w56 w74 w81 w120 w251 w277 w311 w341 w367 w401 w433] -> w28
      tunnel: [w45 w55 w73 w80 w119 w250 w281 w307 w340 w371 w397 w432] -> w27
      tunnel: w26 -> [w46 w56 w74 w81 w117 w251 w277 w311 w341 w367 w401 w433]
      tunnel: w25 -> [w45 w55 w73 w80 w116 w250 w281 w307 w340 w371 w397 w432]
      tunnel: "how much HDI" -> [_ _ _ _ w114 _ _ _ _ _ _ _]
      tunnel: w23 -> [_ _ _ _ w113 _ _ _ _ _ _ _]
      tunnel: w21 -> [w43 w53 w69 w84 w112 w276 w306 w336 w366 w396 w426 w430]
      tunnel: [w43 w53 w68 w84 w112 w276 w306 w336 w366 w396 w426 w430] -> w20
      tunnel: w19 -> [w41 w51 w67 w85 w110 w274 w304 w334 w364 w394 w424 w429]
      tunnel: [w41 w51 w66 w85 w110 w274 w304 w334 w364 w394 w424 w429] -> w18
      tunnel: w17 -> [w42 w52 w65 w86 w111 w273 w303 w333 w363 w393 w423 w428]
      tunnel: [w42 w52 w64 w86 w111 w273 w303 w333 w363 w393 w423 w428] -> w16
      tunnel: [w40 w50 w62 w77 w109 w247 w278 w308 w337 w368 w398 w427] -> w15
      tunnel: w14 -> [w40 w50 w62 _ w109 w247 w278 w308 w337 w368 w398 w427]
      tunnel: 200.0 ("Speed") -> [_ _ _ _ _ w256 w286 w316 w346 w376 w406 _]
      tunnel: 10.0 ("Speed") -> [_ _ _ _ _ w255 w285 w315 w345 w375 w405 _]
      event Timeout {
        n10 = event-data() -> ()  [unwired: 1 in, 3 out]
      }
      event "go to park": Value Change {
        n11 = event-data() -> ()  [unwired: 1 in, 6 out]
        n12 = call "XYZTheta Go.vi"("XYZTheta In"="Parking position", "Motion in"=w60) -> ("Motion out"=w59:refnum<class "Motion.lvclass">)  [unwired: 7 in, 2 out]
      }
      event "calculate": Value Change {
        n13 = event-data() -> ()  [unwired: 1 in, 6 out]
        n14 = Add(x=1.0, y=w69) -> (x+y=w68:dbl)
        n15 = Insert Into Array(array=w65, new element=w62) -> (w64:dbl[][][])  [unwired: 3 in]
        "position from OGP all" <- w64
        n16 = Subtract(x=w71, y=w62) -> (x-y=w63:dbl[][])
        "HDI - stave deviation on time" <- w63
        n17 = Insert Into Array(array=w67, new element=w63) -> (w66:dbl[][][])  [unwired: 3 in]
        "HDI-stave deviation all" <- w66
        "position from OGP on time" <- w62
      }
      event "north first switch": Value Change {
        n18 = event-data() -> ()  [unwired: 1 in, 6 out]
        n19 = flat-sequence {
          tunnel: [w91] -> w78
          tunnel: w78 -> [w106]
          tunnel: [w106] -> w77
          frame #0 {
            n20 = call-poly <vilib>:"Read Delimited Spreadsheet.vi"("file path (dialog if empty)"=path "D:/INTT/V1/Assembly Data/ladder assembly/stave_HDI_center.txt" ("file path (dialog if empty) 3"), "format (%.3f)"="%.8f") -> ("all rows"=w92:dbl[][])  [unwired: 8 in, 5 out]
            n21 = Array Subset(array=w92, index (row)=0 ("index"), length (row)=1 ("length"), index (col)=0 ("index"), length (col)=4 ("length")) -> (w102:dbl[][])
            n22 = Reshape Array(w102, 4 ("dimension size")) -> (w89:dbl[])
            n23 = Array Subset(array=w92, index (row)=1 ("index"), length (row)=1 ("length"), index (col)=0 ("index"), length (col)=4 ("length")) -> (w96:dbl[][])
            n24 = Reshape Array(w96, 4 ("dimension size")) -> (w90:dbl[])
            n25 = Build Array(w90, w89) -> (w91:dbl[][])
          }
          frame #1 {
            n26 = call-poly <vilib>:"Write Delimited Spreadsheet.vi"("file path (dialog if empty)"=path "D:/INTT/V1/Assembly Data/ladder assembly/stave_HDI_center.txt" ("file path (dialog if empty) 4"), "format (%.3f)"="%.8f", "2D data"=w106) -> ()  [unwired: 11 in, 2 out]
          }
        }
      }
      event "measure HDI position": Value Change {
        n27 = event-data() -> ()  [unwired: 1 in, 6 out]
        n28 = Add(x=1.0, y=w130) -> (x+y=w128:dbl)
        "measure times" <- w128
        n29 = Greater?(x=w128, y=1.0) -> (0:w126:bool)
        n30 = Not(x=w126) -> (.not. x?=w125:bool)
        n31 = case shown="False" w125 {
          tunnel: w131 -> [w133 w188]
          tunnel: [w134 w181] -> w115
          tunnel: w124 -> [_ w187]
          tunnel: w123 -> [_ w186]
          tunnel: [w138 w185] -> w122
          tunnel: [w141 w184] -> w121
          tunnel: [w140 w183] -> w120
          tunnel: [w139 w182] -> w119
          tunnel: w118 -> [w137 _]
          tunnel: w117 -> [w136 _]
          tunnel: w116 -> [w135 _]
          tunnel: w114 -> [w132 w180]
          tunnel: w113 -> [_ w179]
          frame False {
            n32 = for {
              N: w132 -> [_]
              shift-right: [w159] -> w134
              shift-left: w133 -> [w160]
              tunnel: [w175] -> _ mode=indexing
              tunnel: [w151] -> w138 mode=indexing
              tunnel: [w150] -> w141 mode=indexing
              tunnel: [w149] -> w140 mode=indexing
              tunnel: [w148] -> w139 mode=indexing
              tunnel: w137 -> [w146] mode=indexing
              tunnel: w136 -> [w144] mode=indexing
              tunnel: w135 -> [w143] mode=indexing
              (unwired) "ideal delta Y between \n2 fiducial marks"
              (unwired) "ideal delta X between 2 fiducial marks"
              # "rotation"
              # "1"
              # "3"
              n33 = call "Joystick and Camera SHIH VPC- external Connection.vi"("Motion in"=w160, "XYZTheta"=w146, "Measurement Point"="Measure Top-Left of HDI", "Inital GO"=TRUE) -> ("Motion out"=w145:refnum<class "Motion.lvclass">, "Sum"=w150:dbl[])  [unwired: 3 in, 2 out]
              n34 = call "Joystick and Camera SHIH VPC- external Connection.vi"("Motion in"=w145, "XYZTheta"=w144, "Measurement Point"="Measure Bottom-Left of HDI", "Inital GO"=TRUE) -> ("Motion out"=w142:refnum<class "Motion.lvclass">, "Sum"=w149:dbl[])  [unwired: 3 in, 2 out]
              n35 = Subtract(x=w149, y=w150) -> (x-y=w168:dbl[])
              n36 = call "XY_to_Rotation_RPHI.vi"("X-Y"=w168) -> ("r-phi"=w164:dbl[])
              n37 = call "Joystick and Camera SHIH VPC- external Connection.vi"("Motion in"=w142, "XYZTheta"=w143, "Measurement Point"="Measure Bottom-Righ of HDI", "Inital GO"=TRUE) -> ("Motion out"=w159:refnum<class "Motion.lvclass">, "Sum"=w148:dbl[])  [unwired: 3 in, 2 out]
              n38 = Subtract(x=w148, y=w150) -> (x-y=w157:dbl[])
              n39 = Index Array(array=w164, index=1) -> (element=w161:dbl)
              n40 = Multiply(x=w161, y=-1.0) -> (x*y=w155:dbl)
              n41 = Replace Array Subset(array=w157, new element=w155, index=3) -> (w175:dbl[])
              n42 = Build Array(24.3 ("y"), 231.4 ("y"), 0.0 ("element"), -0.05 ("element")) -> ()  [unwired: 1 out]
              n43 = Replace Array Subset(array=w150, new element=w155, index=3) -> ()  [unwired: 1 out]
              n44 = Add(x=w148, y=w150) -> (x+y=w177:dbl[])
              n45 = Divide(x=w177, y=2.0) -> (x/y=w154:dbl[])
              n46 = Replace Array Subset(array=w154, new element=w155, index=3) -> (w152:dbl[])
              n47 = Subtract(x=w152, y=dbl[] [0.4, 0.4, 0.0, 0.0]) -> (x-y=w151:dbl[])
            }
          }
          frame True {
            n48 = for {
              N: w180 -> [_]
              tunnel: w187 -> [w209]
              shift-right: [w207] -> w181
              shift-left: w188 -> [w208]
              tunnel: w186 -> [w191]
              tunnel: [w241] -> _ mode=indexing
              tunnel: [w199] -> w185 mode=indexing
              tunnel: [w198] -> w184 mode=indexing
              tunnel: [w197] -> w183 mode=indexing
              tunnel: [w196] -> w182 mode=indexing
              tunnel: w179 -> [w189]
              i -> [w193]
              (unwired) "ideal delta Y between \n2 fiducial marks"
              (unwired) "ideal delta X between 2 fiducial marks"
              # "rotation"
              # "1"
              # "3"
              n49 = Equal?(x=0, y=w193) -> (x = y?=w194:bool)
              n50 = case shown="True" w194 {
                tunnel: [w245 w246] -> w190
                tunnel: w191 -> [_ w246]
                tunnel: w189 -> [w245 _]
                frame False {
                }
                frame True {
                }
              }
              n51 = call "Joystick and Camera SHIH VPC- external Connection.vi"("Motion in"=w208, "XYZTheta"=w190, "Measurement Point"="Measure Top-Left of HDI", "Inital GO"=TRUE) -> ("Motion out"=w221:refnum<class "Motion.lvclass">, "Sum"=w198:dbl[])  [unwired: 3 in, 2 out]
              n52 = Add(x=w209, y=w198) -> (x+y=w225:dbl[])
              n53 = Index Array(array=w198, index=0) -> (element=w212:dbl)
              n54 = Array Subset(array=w225, index=0, length=2) -> (w224:dbl[])
              n55 = Replace Array Subset(array=w224, new element=w212, index=0) -> (w222:dbl[])
              n56 = call-dynamic "XY Go.vi"("Speed"=100.0, "XY"=w222, "Motion in"=w221) -> ("Motion out"=w229:refnum<class "Motion.lvclass">)  [unwired: 7 in, 1 out]
              n57 = call "Joystick and Camera SHIH VPC- external Connection.vi"("Motion in"=w229, "Measurement Point"="Measure Bottom-Left of HDI", "Inital GO"=FALSE) -> ("Motion out"=w220:refnum<class "Motion.lvclass">, "Sum"=w197:dbl[])  [unwired: 4 in, 2 out]
              n58 = Array Subset(array=w225, index=0, length=2) -> (w235:dbl[])
              n59 = Subtract(x=w197, y=w198) -> (x-y=w219:dbl[])
              n60 = call-dynamic "XY Go.vi"("Speed"=100.0, "XY"=w235, "Motion in"=w220) -> ("Motion out"=w239:refnum<class "Motion.lvclass">)  [unwired: 7 in, 1 out]
              n61 = call "XY_to_Rotation_RPHI.vi"("X-Y"=w219) -> ("r-phi"=w215:dbl[])
              n62 = call "Joystick and Camera SHIH VPC- external Connection.vi"("Motion in"=w239, "Measurement Point"="Measure Bottom-Righ of HDI", "Inital GO"=FALSE) -> ("Motion out"=w207:refnum<class "Motion.lvclass">, "Sum"=w196:dbl[])  [unwired: 4 in, 2 out]
              n63 = Subtract(x=w196, y=w198) -> (x-y=w205:dbl[])
              n64 = Index Array(array=w215, index=1) -> (element=w210:dbl)
              n65 = Multiply(x=w210, y=-1.0) -> (x*y=w203:dbl)
              n66 = Replace Array Subset(array=w205, new element=w203, index=3) -> (w241:dbl[])
              n67 = Build Array(24.3 ("y"), 231.4 ("y"), 0.0 ("element"), -0.05 ("element")) -> ()  [unwired: 1 out]
              n68 = Replace Array Subset(array=w198, new element=w203, index=3) -> ()  [unwired: 1 out]
              n69 = Add(x=w196, y=w198) -> (x+y=w243:dbl[])
              n70 = Divide(x=w243, y=2.0) -> (x/y=w202:dbl[])
              n71 = Replace Array Subset(array=w202, new element=w203, index=3) -> (w200:dbl[])
              n72 = Subtract(x=w200, y=dbl[] [0.4, 0.4, 0.0, 0.0]) -> (x-y=w199:dbl[])
            }
          }
        }
      }
      event "north - upper left": Value Change {
        n73 = event-data() -> ()  [unwired: 1 in, 6 out]
        n74 = Array Subset(array=w248, index (row)=0 ("index"), length (row)=1 ("length"), index (col)=0 ("index"), length (col)=4 ("length")) -> (w268:dbl[][])
        n75 = Reshape Array(w268, 4 ("dimension size")) -> (w266:dbl[])
        n76 = Index Array(array=w266, index #1=0 ("index"), index #2=1 ("index"), index #3=2 ("index")) -> (element #1=w262:dbl, element #2=w261:dbl, element #3=w259:dbl)
        n77 = Build Array(w262, w261) -> (w260:dbl[])
        n78 = call-dynamic "XY Go.vi"("Speed"=w256, "XY"=w260, "Motion in"=w257) -> ("Motion out"=w258:refnum<class "Motion.lvclass">)  [unwired: 7 in, 1 out]
        n79 = call-dynamic "Z Go.vi"("Speed"=w255, "Position"=w259, "Motion in"=w258) -> ("Motion out"=w254:refnum<class "Motion.lvclass">)  [unwired: 7 in, 1 out]
        n80 = call "Joystick and Camera SHIH VPC- external Connection.vi"("Motion in"=w254, "Inital GO"=FALSE) -> ("Motion out"=w252:refnum<class "Motion.lvclass">)  [unwired: 5 in, 3 out]
      }
      event "north - bottom left": Value Change {
        n81 = event-data() -> ()  [unwired: 1 in, 6 out]
        n82 = Array Subset(array=w277, index (row)=0 ("index"), length (row)=1 ("length"), index (col)=0 ("index"), length (col)=4 ("length")) -> (w298:dbl[][])
        n83 = Reshape Array(w298, 4 ("dimension size")) -> (w296:dbl[])
        n84 = Index Array(array=w296, index #1=0 ("index"), index #2=1 ("index"), index #3=2 ("index")) -> (element #1=w292:dbl, element #2=w291:dbl, element #3=w289:dbl)
        n85 = Build Array(w292, w291) -> (w290:dbl[])
        n86 = call-dynamic "XY Go.vi"("Speed"=w286, "XY"=w290, "Motion in"=w287) -> ("Motion out"=w288:refnum<class "Motion.lvclass">)  [unwired: 7 in, 1 out]
        n87 = call-dynamic "Z Go.vi"("Speed"=w285, "Position"=w289, "Motion in"=w288) -> ("Motion out"=w284:refnum<class "Motion.lvclass">)  [unwired: 7 in, 1 out]
        n88 = call "Joystick and Camera SHIH VPC- external Connection.vi"("Motion in"=w284, "Inital GO"=FALSE) -> ("Motion out"=w282:refnum<class "Motion.lvclass">)  [unwired: 5 in, 3 out]
      }
      event "north - bottom right": Value Change {
        n89 = event-data() -> ()  [unwired: 1 in, 6 out]
        n90 = Array Subset(array=w307, index (row)=0 ("index"), length (row)=1 ("length"), index (col)=0 ("index"), length (col)=4 ("length")) -> (w328:dbl[][])
        n91 = Reshape Array(w328, 4 ("dimension size")) -> (w326:dbl[])
        n92 = Index Array(array=w326, index #1=0 ("index"), index #2=1 ("index"), index #3=2 ("index")) -> (element #1=w322:dbl, element #2=w321:dbl, element #3=w319:dbl)
        n93 = Build Array(w322, w321) -> (w320:dbl[])
        n94 = call-dynamic "XY Go.vi"("Speed"=w316, "XY"=w320, "Motion in"=w317) -> ("Motion out"=w318:refnum<class "Motion.lvclass">)  [unwired: 7 in, 1 out]
        n95 = call-dynamic "Z Go.vi"("Speed"=w315, "Position"=w319, "Motion in"=w318) -> ("Motion out"=w314:refnum<class "Motion.lvclass">)  [unwired: 7 in, 1 out]
        n96 = call "Joystick and Camera SHIH VPC- external Connection.vi"("Motion in"=w314, "Inital GO"=FALSE) -> ("Motion out"=w312:refnum<class "Motion.lvclass">)  [unwired: 5 in, 3 out]
      }
      event "south - upper left": Value Change {
        n97 = event-data() -> ()  [unwired: 1 in, 6 out]
        n98 = Array Subset(array=w338, index (row)=1 ("index"), length (row)=1 ("length"), index (col)=0 ("index"), length (col)=4 ("length")) -> (w358:dbl[][])
        n99 = Reshape Array(w358, 4 ("dimension size")) -> (w356:dbl[])
        n100 = Index Array(array=w356, index #1=0 ("index"), index #2=1 ("index"), index #3=2 ("index")) -> (element #1=w352:dbl, element #2=w351:dbl, element #3=w349:dbl)
        n101 = Build Array(w352, w351) -> (w350:dbl[])
        n102 = call-dynamic "XY Go.vi"("Speed"=w346, "XY"=w350, "Motion in"=w347) -> ("Motion out"=w348:refnum<class "Motion.lvclass">)  [unwired: 7 in, 1 out]
        n103 = call-dynamic "Z Go.vi"("Speed"=w345, "Position"=w349, "Motion in"=w348) -> ("Motion out"=w344:refnum<class "Motion.lvclass">)  [unwired: 7 in, 1 out]
        n104 = call "Joystick and Camera SHIH VPC- external Connection.vi"("Motion in"=w344, "Inital GO"=FALSE) -> ("Motion out"=w342:refnum<class "Motion.lvclass">)  [unwired: 5 in, 3 out]
      }
      event "south - bottom left": Value Change {
        n105 = event-data() -> ()  [unwired: 1 in, 6 out]
        n106 = Array Subset(array=w367, index (row)=1 ("index"), length (row)=1 ("length"), index (col)=0 ("index"), length (col)=4 ("length")) -> (w388:dbl[][])
        n107 = Reshape Array(w388, 4 ("dimension size")) -> (w386:dbl[])
        n108 = Index Array(array=w386, index #1=0 ("index"), index #2=1 ("index"), index #3=2 ("index")) -> (element #1=w382:dbl, element #2=w381:dbl, element #3=w379:dbl)
        n109 = Build Array(w382, w381) -> (w380:dbl[])
        n110 = call-dynamic "XY Go.vi"("Speed"=w376, "XY"=w380, "Motion in"=w377) -> ("Motion out"=w378:refnum<class "Motion.lvclass">)  [unwired: 7 in, 1 out]
        n111 = call-dynamic "Z Go.vi"("Speed"=w375, "Position"=w379, "Motion in"=w378) -> ("Motion out"=w374:refnum<class "Motion.lvclass">)  [unwired: 7 in, 1 out]
        n112 = call "Joystick and Camera SHIH VPC- external Connection.vi"("Motion in"=w374, "Inital GO"=FALSE) -> ("Motion out"=w372:refnum<class "Motion.lvclass">)  [unwired: 5 in, 3 out]
      }
      event "south - bottom right": Value Change {
        n113 = event-data() -> ()  [unwired: 1 in, 6 out]
        n114 = Array Subset(array=w397, index (row)=1 ("index"), length (row)=1 ("length"), index (col)=0 ("index"), length (col)=4 ("length")) -> (w418:dbl[][])
        n115 = Reshape Array(w418, 4 ("dimension size")) -> (w416:dbl[])
        n116 = Index Array(array=w416, index #1=0 ("index"), index #2=1 ("index"), index #3=2 ("index")) -> (element #1=w412:dbl, element #2=w411:dbl, element #3=w409:dbl)
        n117 = Build Array(w412, w411) -> (w410:dbl[])
        n118 = call-dynamic "XY Go.vi"("Speed"=w406, "XY"=w410, "Motion in"=w407) -> ("Motion out"=w408:refnum<class "Motion.lvclass">)  [unwired: 7 in, 1 out]
        n119 = call-dynamic "Z Go.vi"("Speed"=w405, "Position"=w409, "Motion in"=w408) -> ("Motion out"=w404:refnum<class "Motion.lvclass">)  [unwired: 7 in, 1 out]
        n120 = call "Joystick and Camera SHIH VPC- external Connection.vi"("Motion in"=w404, "Inital GO"=FALSE) -> ("Motion out"=w402:refnum<class "Motion.lvclass">)  [unwired: 5 in, 3 out]
      }
      event "test": Value Change {
        n121 = event-data() -> ()  [unwired: 1 in, 6 out]
        n122 = Equal?(x=0.0, y=0.0) -> (x = y?=w435:bool)
        n123 = case shown="True" w435 {
          tunnel: w441 -> [w442 w446]
          tunnel: [w442 w445] -> w440
          tunnel: w438 -> [_ w444]
          frame False {
          }
          frame True {
            n124 = for {
              N: 2 -> [_]
              tunnel: w444 -> [w448]
              shift-right: [w449] -> w445
              shift-left: w446 -> [w450]
              n125 = call "Joystick and Camera SHIH VPC- external Connection.vi"("Motion in"=w450, "XYZTheta"=w448, "Inital GO"=TRUE) -> ("Motion out"=w449:refnum<class "Motion.lvclass">)  [unwired: 4 in, 3 out]
            }
          }
        }
      }
    }
    n126 = feedback-in #1(w30) -> ()
    n127 = feedback-in #2(w28) -> ()
    n128 = feedback-in #3(w27) -> ()
    n129 = feedback-in #4(w15) -> ()
    n130 = feedback-in #5(w31) -> ()
  }
  n131 = call-dynamic "Disconnect.vi"("Controller in"=w8) -> ()  [unwired: 9 in, 1 out]
